vi "ProgrämmschenEinfacherEditor.vi"() -> ()   [LabVIEW 2010]
uses:
  <vilib>/userDefined/High Color/nirio_resource_hc.ctl
  <vilib>/rvi/interface/nirviOpenFPGA/nirviOpenFPGA.xnode
  C:/Users/HAGAR-IV/Desktop/Zeugs/markus/version feb 2012/test/Auslesenkopiekopie2.vi
  <vilib>/rvi/interface/nirviMethod/nirviMethod.xnode
  <vilib>/rvi/interface/nirviReadWriteControl/nirviReadWriteControl.xnode
  <vilib>/rvi/errors/niLvFpgaWhatHappensToTopLevelVI.ctl
  <vilib>/rvi/interface/common/niFpgaNodeNameForErrorReporting.ctl
  <vilib>/rvi/errors/niLvFpgaAdjustHostInterfaceError.vi
  gvbooleschRT.vi
  <vilib>/functionblocks/FB Core/FB Core.xnode
  <vilib>/functionblocks/Counter/Elapsed Timer/Elapsed Timer.vi
  <vilib>/functionblocks/NI_FunctionBlock Libraries.lvlib
  <vilib>/rvi/interface/nirviCloseFPGA/nirviCloseFPGA.xnode
  <vilib>/addons/control/pid/NI_PID_pid.lvlib
  <vilib>/addons/control/pid/pid.llb/PID (DBL).vi
  <vilib>/LabVIEW Targets/FPGA/cRIO/shared/nicrio_ModuleControls/nicrio_cRIO-9871_BaudRateEnum.ctl
  <vilib>/LabVIEW Targets/FPGA/cRIO/shared/nicrio_ModuleControls/nicrio_cRIO-9871_DataBitsEnum.ctl
  <vilib>/LabVIEW Targets/FPGA/cRIO/shared/nicrio_ModuleControls/nicrio_cRIO-9871_ParityEnum.ctl
  <vilib>/LabVIEW Targets/FPGA/cRIO/shared/nicrio_ModuleControls/nicrio_cRIO-9871_StopBitsEnum.ctl
  <vilib>/LabVIEW Targets/FPGA/cRIO/shared/nicrio_ModuleControls/nicrio_cRIO-9871_FlowControlEnum.ctl
  <vilib>/addons/internet/NI_InternetTK_FTP_VIs.lvlib
  <vilib>/RVI Host/nirviSupport.llb/nirviErrorClusterFromErrorCode.vi
  <vilib>/FPGAPlugInAG/cRIO-9114/niLvFpga_Close_cRIO-9114.vi
panel:
  in  "dargestellte Größe 2":i32(ring)=1 items=["T-MainCol3", "T-Trap1", "T-Trap2", "T-Stirling", "T-PreCol1", "T-PreCol2", "T-MainCol1", "T-MainCol2", "T-T-Line2", "T-MI1", "T-MI2", "T-MI3", "T-MI4", "T-MI5", "T-MI6", "F-MFM1", "T-MainCol4", "T-BHorst1", "T-BHorst2", "T-BHorst3", "T-BHorst4", "T-Oven1", "T-Oven2", "T-T-Line1", "F-MFM2", "P-Me-HP", "P-Me-LP", "P-Vac", "Ref-Turbo", "I-MS-AC", "I-Trap1", "I-Trap2", "Mod2/AI0", "Mod2/AI1", "Mod2/AI2", "Mod2/AI3", "Mod2/AI4", "Mod2/AI5", "Mod2/AI6", "Mod2/AI7", "Mod2/AI8", "Mod2/AI9", "Mod2/AI10", "Mod2/AI11", "Mod2/AI12", "Mod2/AI13", "Mod2/AI14", "Mod2/AI15", "Mod2/AI16", "Mod2/AI17", "Mod2/AI18", "Mod2/AI19", "Mod2/AI20", "Mod2/AI21", "Mod2/AI22", "Mod2/AI23", "Mod2/AI24", "Mod2/AI25", "Mod2/AI26", "Mod2/AI27", "Mod2/AI28", "Mod2/AI29", "Mod2/AI30", "Mod2/AI31", "Mod3/AI0", "Mod3/AI1", "Mod3/AI2", "Mod3/AI3", "Mod3/AI4", "Mod3/AI5", "Mod3/AI6", "Mod3/AI7", "Mod3/AI8", "Mod3/AI9", "Mod3/AI10", "Mod3/AI11", "Mod3/AI12", "Mod3/AI13", "Mod3/AI14", "Mod3/AI15", "Mod3/AI16", "Mod3/AI17", "Mod3/AI18", "Mod3/AI19", "Mod3/AI20", "Mod3/AI21", "Mod3/AI22", "Mod3/AI23", "Mod3/AI24", "Mod3/AI25", "Mod3/AI26", "Mod3/AI27", "Mod3/AI28", "Mod3/AI29", "Mod3/AI30", "Mod3/AI31", "U_Widr.Trap1 [V]", "Temp.Trap1 [°C]", "U_Widr.Trap2 [V]", "Temp.Trap2 [°C]", "Temp.Mach1 [°C]", "Temp.Mach2 [°C]", "MFC1B", "PressContr1A", "PressContr1B", "PressContr1C", "MFC1A", "PressContr1D"]
  in  "Zeitachse2":i32(ring)=1 items=["Zykluszeit [s] Mod0", "Zykluszeit [s] Mod1", "Zykluszeit [s] Mod2A", "Zykluszeit [s] Mod2B"]
  out "Anzeige2":cluster{dbl[], dbl[]}(graph)
  out "Datum/Zeit":string
  in  "wie wird gespeichert?":u16(ring) items=["Time", "Cycle", "All"]
  out "Text 6":string
  in  "Info":string
  in  "Speicherlänge":string
  in  "Dateien fürs MS schicken?":bool
  in  "Pfad MS-Datei CRIO":path
  in  "Text0 MS-Datei":string
  out "ZwangsHorst!":cluster{dbl[]}[](array[cluster])
  out "ZwangsHorst?":cluster{bool[]}[](array[cluster])
  out "ZwangsDIO!":cluster{bool[]}[](array[cluster])
  out "ZwangsDIO?":cluster{bool[]}[](array[cluster])
  out "PIDs für \"träge\" Heizungen":T1(array[cluster])
  out "ZwangsLangsameH!":bool[](array[boolean])
  in  "Heizen?LH":bool[](array[boolean])
  out "Zwangsbedingungen":dbl[][](array[numeric])
  out "Traps/Machs":dbl[](array[numeric])
  out "ZwangsFPGABoolesch!":bool[](array[boolean])
  out "ZwangsFPGABoolesch?":bool[](array[boolean])
  in  "LangsameHeizungen%":u32[](array[numeric])
  in  "LangsameHeizungenSP":dbl[](array[numeric])
  out "ZwangsLangsameH?":bool[](array[boolean])
  out "Zykluszeiten 0, 1, 2A, 2B":dbl[](array[numeric])
  out "Zyklusnummern 0, 1, 2A, 2B":i32[](array[numeric])
  in  "dargestellte Größe 1":i32(ring)=1 items=["T-MainCol3", "T-Trap1", "T-Trap2", "T-Stirling", "T-PreCol1", "T-PreCol2", "T-MainCol1", "T-MainCol2", "T-T-Line2", "T-MI1", "T-MI2", "T-MI3", "T-MI4", "T-MI5", "T-MI6", "F-MFM1", "T-MainCol4", "T-BHorst1", "T-BHorst2", "T-BHorst3", "T-BHorst4", "T-Oven1", "T-Oven2", "T-T-Line1", "F-MFM2", "P-Me-HP", "P-Me-LP", "P-Vac", "Ref-Turbo", "I-MS-AC", "I-Trap1", "I-Trap2", "Mod2/AI0", "Mod2/AI1", "Mod2/AI2", "Mod2/AI3", "Mod2/AI4", "Mod2/AI5", "Mod2/AI6", "Mod2/AI7", "Mod2/AI8", "Mod2/AI9", "Mod2/AI10", "Mod2/AI11", "Mod2/AI12", "Mod2/AI13", "Mod2/AI14", "Mod2/AI15", "Mod2/AI16", "Mod2/AI17", "Mod2/AI18", "Mod2/AI19", "Mod2/AI20", "Mod2/AI21", "Mod2/AI22", "Mod2/AI23", "Mod2/AI24", "Mod2/AI25", "Mod2/AI26", "Mod2/AI27", "Mod2/AI28", "Mod2/AI29", "Mod2/AI30", "Mod2/AI31", "Mod3/AI0", "Mod3/AI1", "Mod3/AI2", "Mod3/AI3", "Mod3/AI4", "Mod3/AI5", "Mod3/AI6", "Mod3/AI7", "Mod3/AI8", "Mod3/AI9", "Mod3/AI10", "Mod3/AI11", "Mod3/AI12", "Mod3/AI13", "Mod3/AI14", "Mod3/AI15", "Mod3/AI16", "Mod3/AI17", "Mod3/AI18", "Mod3/AI19", "Mod3/AI20", "Mod3/AI21", "Mod3/AI22", "Mod3/AI23", "Mod3/AI24", "Mod3/AI25", "Mod3/AI26", "Mod3/AI27", "Mod3/AI28", "Mod3/AI29", "Mod3/AI30", "Mod3/AI31", "U_Widr.Trap1 [V]", "Temp.Trap1 [°C]", "U_Widr.Trap2 [V]", "Temp.Trap2 [°C]", "Temp.Mach1 [°C]", "Temp.Mach2 [°C]", "MFC1B", "PressContr1A", "PressContr1B", "PressContr1C", "MFC1A", "PressContr1D"]
  in  "Zeitachse1":i32(ring)=1 items=["Zykluszeit [s] Mod0", "Zykluszeit [s] Mod1", "Zykluszeit [s] Mod2A", "Zykluszeit [s] Mod2B"]
  out "Anzeige1":cluster{dbl[], dbl[]}(graph)
  out "Big Ben, Methodenzeit, Zykluszeit0, Zykluszeit1, Zykluszeit2A, Zykluszeit2B":dbl[](array[numeric])
  out "MWHorst":dbl[](array[numeric])
  out "HorstSP":dbl[](array[numeric])
  out "RS-232":string
  out "Port5":string
  out "Zähler serielle Kommunikation":i32
  out "Port6":string
  out "Port7":string
  out "Port8":string
  out "Mod1Mod2Mod3/AITrapsMachs1Hz":dbl[](array[numeric])
  out "Mod3/AI":dbl[](array[numeric])
  out "Mod2/AI":dbl[](array[numeric])
  out "Mod1/AI":dbl[](array[numeric])
  in  "global stop RT":bool
  out "Big Ben":dbl
  out "Methodenzeit":dbl
  out "Zyklnum1ges":i32
  out "aktuelle TDMS-Datei":refnum<k34>
  in  "Methodennummer":i32(ring) items=["0"]
  out "Methodenwechsel?":bool
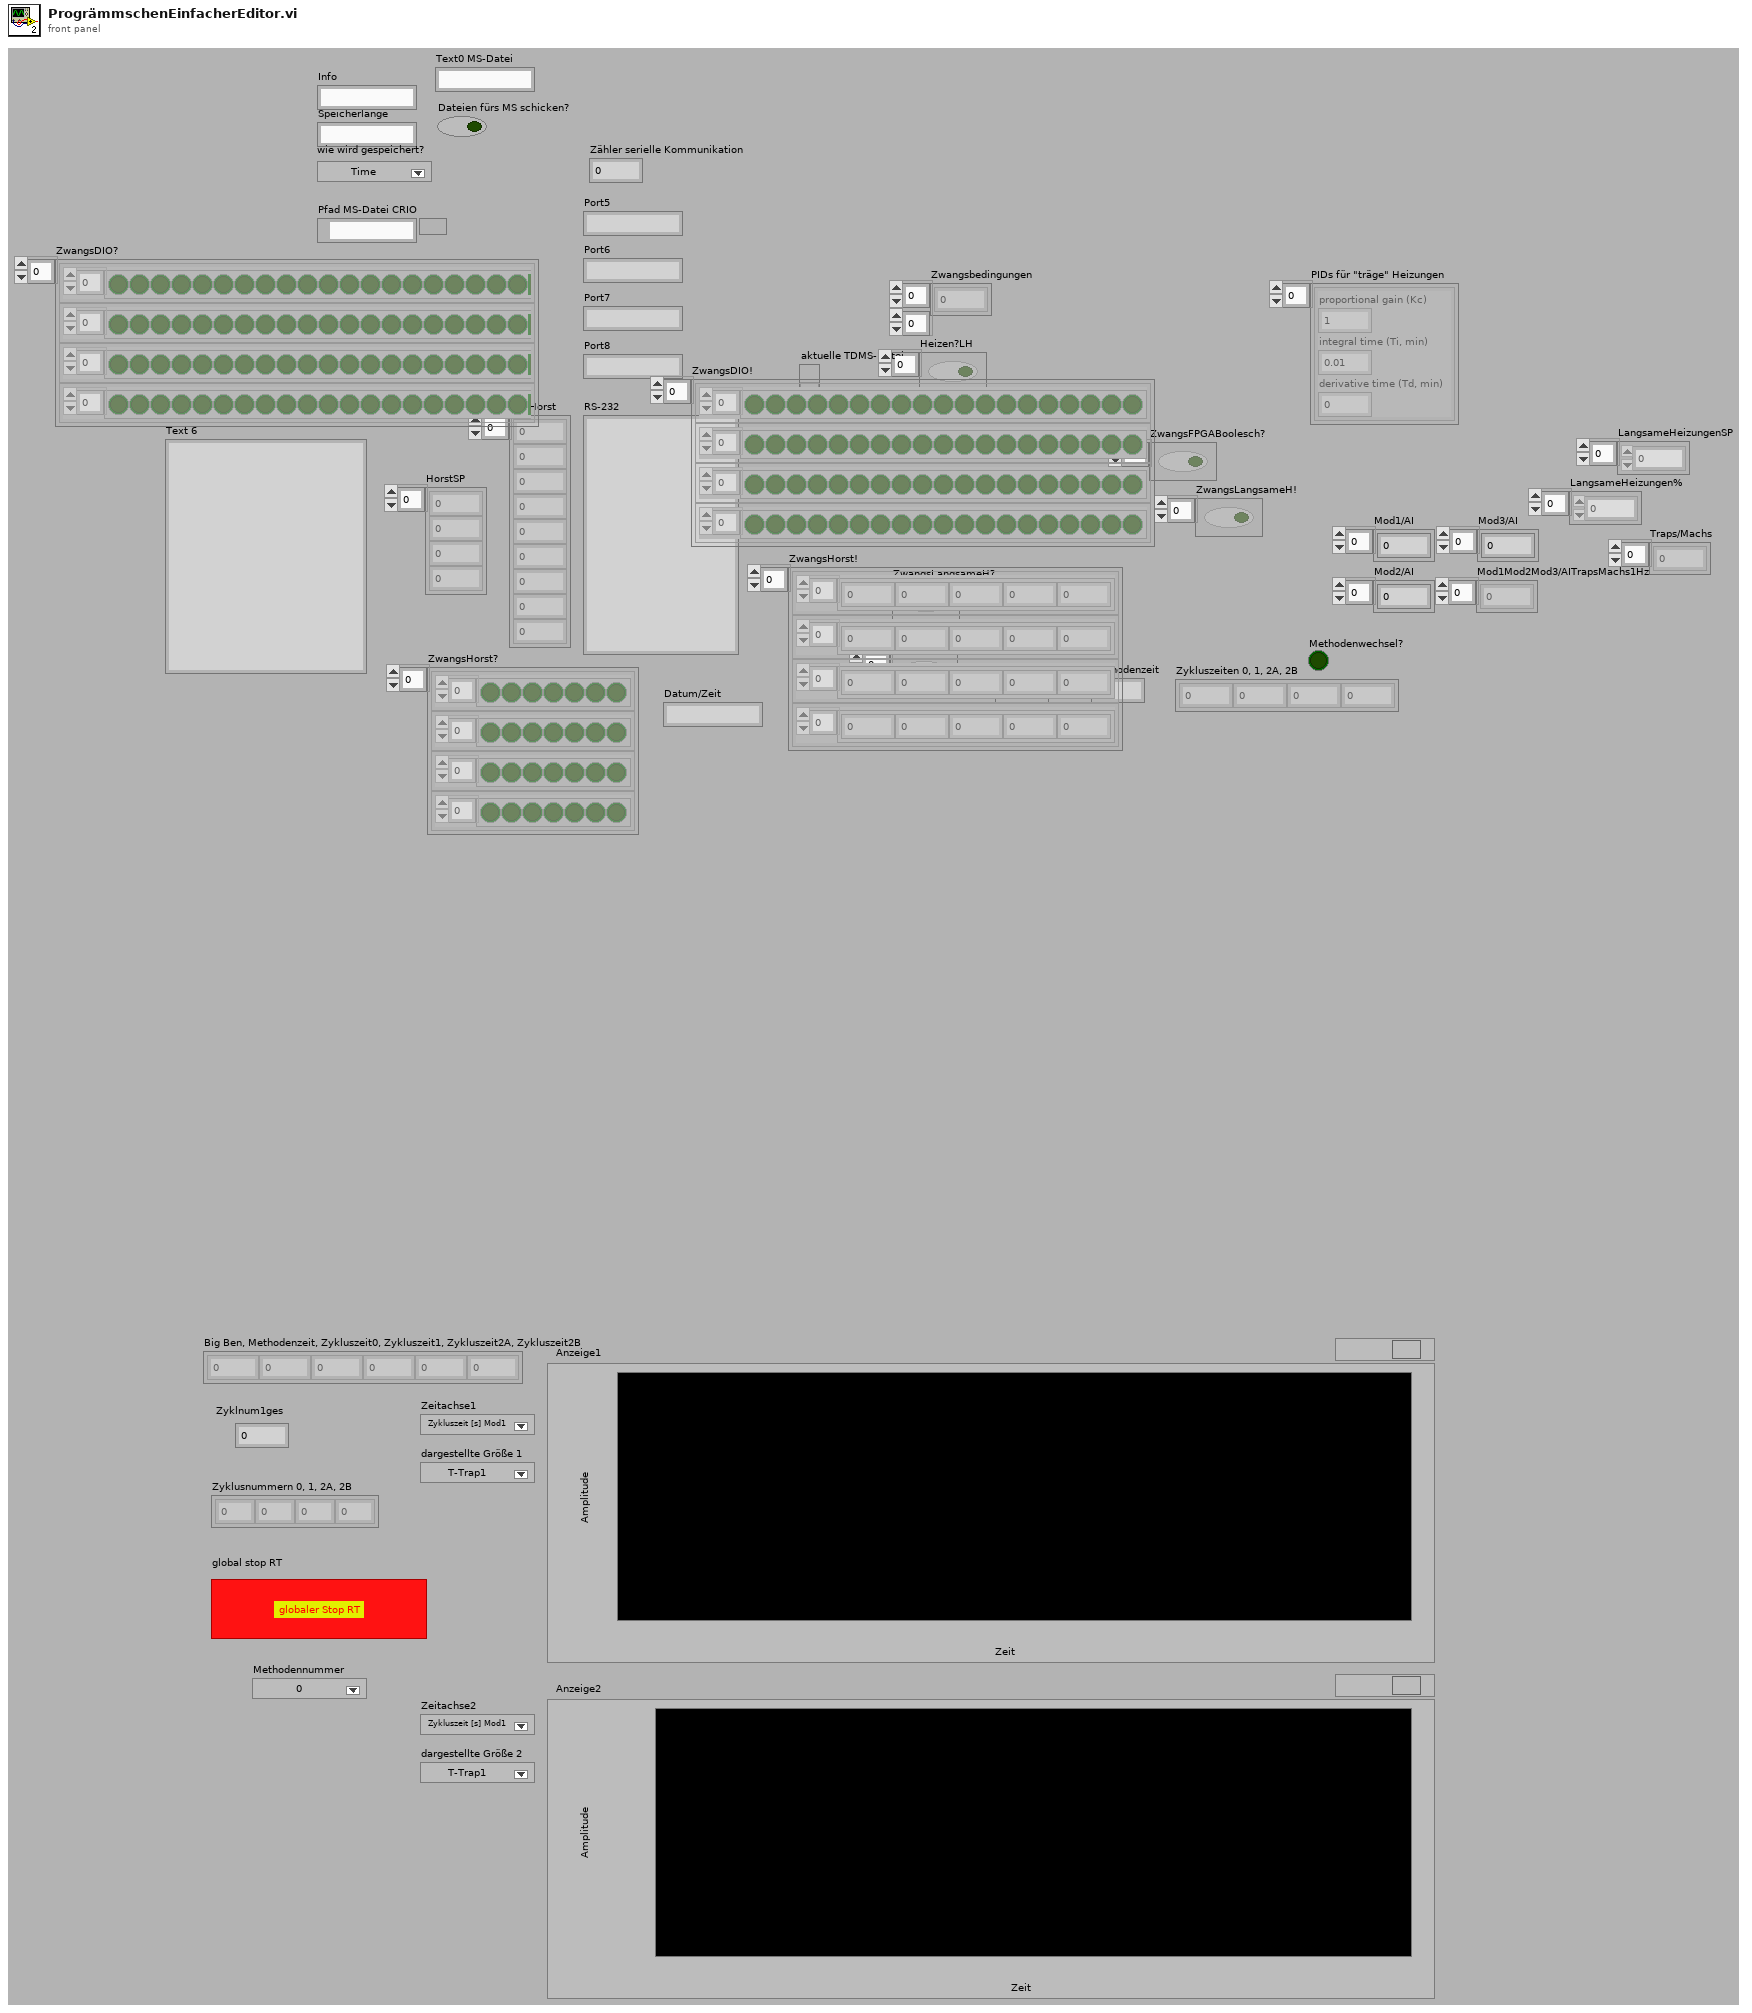
[diagram p1: front panel]
types:
  T1 = cluster{"proportional gain (Kc)":dbl, "integral time (Ti, min)":dbl, "derivative time (Td, min)":dbl}[]
  T2 = cluster{"Zykluslängen [s]":dbl[], "ZeitpktDIOsMod0":dbl[], "ZeitpktDIOsMod1":dbl[], "ZeitpktDIOsMod2A":dbl[], "ZeitpktDIOsMod2B":dbl[], "DIOsSPMod0":bool[][], "DIOsSPMod1":bool[][], "DIOsSPMod2A":bool[][], "DIOsSPMod2B":bool[][], "Mod0HorstZeitpkt":dbl[], "Mod1HorstZeitpkt":dbl[], "Mod2AHorstZeitpkt":dbl[], "Mod2BHorstZeitpkt":dbl[], "HorstSPMod0":dbl[][], "HorstSPMod1":dbl[][], "HorstSPMod2A":dbl[][], "HorstSPMod2B":dbl[][], "LangsameHeizungenSP":dbl[], "LHHeizen?":bool[], "ZPktFPGABoolesch":dbl[], "FPGABoolesch":bool[][], "ZeitpktFPGAPID":dbl[], "FPGAPID":cluster{"proportional gain (Kc)":fxp<+/-,16,8>, "integral gain (Kc*Ts/Ti)":fxp<+/-,16,8>, "derivative gain (Kc*Td/Ts)":fxp<+/-,16,8>}[][], "ZeitpktFPGAFixp":dbl[], "FPGAFixp":fxp<+/-,16,4>[][], "ZeitpktMach1":dbl[], "TempMach1":dbl[], "ZeitpktMach2":dbl[], "TempMach2":dbl[], "PIDs für \"träge\" Heizungen":cluster{"proportional gain (Kc)":dbl, "integral time (Ti, min)":dbl, "derivative time (Td, min)":dbl}[], "Zwangsbedingungen":dbl[][], "Text0 MS-Datei":string, "Info":string, "wie wird gespeichert?":u16, "Speicherlänge":string, "Dateien fürs MS schicken?":bool, "Pfad MS-Datei CRIO":path}[]
  T3 = cluster{"DIOsMod0Nr":i32[], "DIOsMod1Nr":i32[], "DIOsMod2ANr":i32[], "DIOsMod2BNr":i32[], "AIs für \"träge\" Heizungen":i32[], i32[], "AnschlüsseHorstMod0":enum8{"0", "1", "2", "3", "4", "5", "6", "7", "8"}[], "AnschlüsseHorstMod1":enum8{"0", "1", "2", "3", "4", "5", "6", "7", "8"}[], "AnschlüsseHorstMod2A":enum8{"0", "1", "2", "3", "4", "5", "6", "7", "8"}[], "AnschlüsseHorstMod2B":enum8{"0", "1", "2", "3", "4", "5", "6", "7", "8"}[], "StringSPvorgebenMod0":string[], "StringSPvorgebenMod1":string[], "StringSPvorgebenMod2A":string[], "StringSPvorgebenMod2B":string[], "StringMWAntwort0":string[], "StringMWAntwort1":string[], "StringMWAntwort2A":string[], "StringMWAntwort2B":string[], "UmrechnungHorst0":dbl[], "UmrechnungHorst1":dbl[], "UmrechnungHorst2A":dbl[], "UmrechnungHorst2B":dbl[], "StringMWabfragenMod0":string[], "StringMWabfragenMod1":string[], "StringMWabfragenMod2A":string[], "StringMWabfragenMod2B":string[], "Modul1/AI koeff":dbl[][], "Modul2/AI koeff":dbl[][], "Modul3/AI koeff":dbl[][], "Traps/MachKoeff":dbl[][], "AIsNamen":string[], "DIOsMod0Name":string[], "DIOsMod1Name":string[], "DIOsMod2AName":string[], "DIOsMod2BName":string[], "HorstMod0Name":string[], "HorstMod1Name":string[], "HorstMod2AName":string[], "HorstMod2BName":string[], "Startmethode":i32, "Dateiordner Housekeeping":path, "Dateiname Housekeeping":string}
  T4 = enum16{"open", "open or create", "create or replace", "create", "open (read-only)"}
  T5 = enum16{"open", "replace", "create", "open or create", "replace or create", "replace or create with confirmation"}
  T6 = typedef "niFpgaNodeNameForErrorReporting.ctl" = enum16{"Open FPGA VI Reference", "Read/Write Control", "Invoke Method: Abort", "Invoke Method: Acknowledge IRQ", "Invoke Method: Download", "Invoke Method: FIFO.Configure", "Invoke Method: FIFO.Read", "Invoke Method: FIFO.Start", "Invoke Method: FIFO.Stop", "Invoke Method: FIFO.Write", "Invoke Method: Reset", "Invoke Method: Run", "Invoke Method: Wait on IRQ", "Close FPGA VI Reference"}
  T7 = typedef "niLvFpgaWhatHappensToTopLevelVI.ctl" = enum16{"top level VI scripted behind XNode", "top level VI inlined behind XNode"}
  T8 = typedef "nicrio_cRIO-9871_BaudRateEnum.ctl" = enum16{"75 bps", "110 bps", "134 bps", "150 bps", "300 bps", "600 bps", "1200 bps", "1800 bps", "2400 bps", "4800 bps", "7200 bps", "9600 bps", "14.4 kbps", "19.2 kbps", "28.8 kbps", "38.4 kbps", "57.6 kbps", "115.2 kbps", "230.4 kbps", "460.8 kbps", "921.6 kbps"}
  T9 = typedef "nicrio_cRIO-9871_DataBitsEnum.ctl" = enum8{"5", "6", "7", "8"}
  T10 = typedef "nicrio_cRIO-9871_ParityEnum.ctl" = enum8{"None", "Odd", "Even", "Mark", "Space"}
  T11 = typedef "nicrio_cRIO-9871_StopBitsEnum.ctl" = enum8{"1", "1.5", "2"}
  T12 = typedef "nicrio_cRIO-9871_FlowControlEnum.ctl" = enum8{"None", "Software (XON / XOFF)", "Hardware (RTS / CTS)"}
  T13 = cluster{"Baud Rate":T8, "Data Bits":T9, "Parity":T10, "Stop Bits":T11, "Flow Control":T12}
  T14 = enum8{"0", "1", "2", "3", "4", "5", "6", "7", "8"}[]
  T15 = cluster{"Heizen?LH[0]":bool, "Heizen?LH[1]":bool, "Heizen?LH[2]":bool, "Heizen?LH[3]":bool, "Heizen?LH[4]":bool, "Heizen?LH[5]":bool}
  T16 = cluster{"LangsameHeizungen%[0]":u32, "LangsameHeizungen%[1]":u32, "LangsameHeizungen%[2]":u32, "LangsameHeizungen%[3]":u32, "LangsameHeizungen%[4]":u32, "LangsameHeizungen%[5]":u32}
  T17 = cluster{"PIDs für \"träge\" Heizungen[0]":cluster{"proportional gain (Kc)":dbl, "integral time (Ti, min)":dbl, "derivative time (Td, min)":dbl}, "PIDs für \"träge\" Heizungen[1]":cluster{"proportional gain (Kc)":dbl, "integral time (Ti, min)":dbl, "derivative time (Td, min)":dbl}, "PIDs für \"träge\" Heizungen[2]":cluster{"proportional gain (Kc)":dbl, "integral time (Ti, min)":dbl, "derivative time (Td, min)":dbl}, "PIDs für \"träge\" Heizungen[3]":cluster{"proportional gain (Kc)":dbl, "integral time (Ti, min)":dbl, "derivative time (Td, min)":dbl}, "PIDs für \"träge\" Heizungen[4]":cluster{"proportional gain (Kc)":dbl, "integral time (Ti, min)":dbl, "derivative time (Td, min)":dbl}, "PIDs für \"träge\" Heizungen[5]":cluster{"proportional gain (Kc)":dbl, "integral time (Ti, min)":dbl, "derivative time (Td, min)":dbl}}
  T18 = cluster{"LangsameHeizungenSP[0]":dbl, "LangsameHeizungenSP[1]":dbl, "LangsameHeizungenSP[2]":dbl, "LangsameHeizungenSP[3]":dbl, "LangsameHeizungenSP[4]":dbl, "LangsameHeizungenSP[5]":dbl}
  T19 = cluster{"[0]":dbl, "[1]":dbl, "[2]":dbl, "[3]":dbl, "[4]":dbl, "[5]":dbl}
  T20 = cluster{"proportional gain (Kc)":dbl, "integral time (Ti, min)":dbl, "derivative time (Td, min)":dbl}
  T21 = cluster{"Zykluslängen [s]":dbl[], "ZeitpktDIOsMod0":dbl[], "ZeitpktDIOsMod1":dbl[], "ZeitpktDIOsMod2A":dbl[], "ZeitpktDIOsMod2B":dbl[], "DIOsSPMod0":bool[][], "DIOsSPMod1":bool[][], "DIOsSPMod2A":bool[][], "DIOsSPMod2B":bool[][], "Mod0HorstZeitpkt":dbl[], "Mod1HorstZeitpkt":dbl[], "Mod2AHorstZeitpkt":dbl[], "Mod2BHorstZeitpkt":dbl[], "HorstSPMod0":dbl[][], "HorstSPMod1":dbl[][], "HorstSPMod2A":dbl[][], "HorstSPMod2B":dbl[][], "LangsameHeizungenSP":dbl[], "LHHeizen?":bool[], "ZPktFPGABoolesch":dbl[], "FPGABoolesch":bool[][], "ZeitpktFPGAPID":dbl[], "FPGAPID":cluster{"proportional gain (Kc)":fxp<+/-,16,8>, "integral gain (Kc*Ts/Ti)":fxp<+/-,16,8>, "derivative gain (Kc*Td/Ts)":fxp<+/-,16,8>}[][], "ZeitpktFPGAFixp":dbl[], "FPGAFixp":fxp<+/-,16,4>[][], "ZeitpktMach1":dbl[], "TempMach1":dbl[], "ZeitpktMach2":dbl[], "TempMach2":dbl[], "PIDs für \"träge\" Heizungen":cluster{"proportional gain (Kc)":dbl, "integral time (Ti, min)":dbl, "derivative time (Td, min)":dbl}[], "Zwangsbedingungen":dbl[][], "Text0 MS-Datei":string, "Info":string, "wie wird gespeichert?":u16, "Speicherlänge":string, "Dateien fürs MS schicken?":bool, "Pfad MS-Datei CRIO":path}
  T22 = cluster{"proportional gain (Kc)":fxp<+/-,16,8>, "integral gain (Kc*Ts/Ti)":fxp<+/-,16,8>, "derivative gain (Kc*Td/Ts)":fxp<+/-,16,8>}[][]
  T23 = cluster{"FPGAFixp[0]":fxp<+/-,16,4>, "FPGAFixp[1]":fxp<+/-,16,4>, "FPGAFixp[2]":fxp<+/-,16,4>, "FPGAFixp[3]":fxp<+/-,16,4>, "FPGAFixp[4]":fxp<+/-,16,4>, "FPGAFixp[5]":fxp<+/-,16,4>, "FPGAFixp[6]":fxp<+/-,16,4>, "FPGAFixp[7]":fxp<+/-,16,4>}
  T24 = cluster{"proportional gain (Kc)":fxp<+/-,16,8>, "integral gain (Kc*Ts/Ti)":fxp<+/-,16,8>, "derivative gain (Kc*Td/Ts)":fxp<+/-,16,8>}[]
  T25 = cluster{"FPGAPID[0]":cluster{"proportional gain (Kc)":fxp<+/-,16,8>, "integral gain (Kc*Ts/Ti)":fxp<+/-,16,8>, "derivative gain (Kc*Td/Ts)":fxp<+/-,16,8>}, "FPGAPID[1]":cluster{"proportional gain (Kc)":fxp<+/-,16,8>, "integral gain (Kc*Ts/Ti)":fxp<+/-,16,8>, "derivative gain (Kc*Td/Ts)":fxp<+/-,16,8>}, "FPGAPID[2]":cluster{"proportional gain (Kc)":fxp<+/-,16,8>, "integral gain (Kc*Ts/Ti)":fxp<+/-,16,8>, "derivative gain (Kc*Td/Ts)":fxp<+/-,16,8>}, "FPGAPID[3]":cluster{"proportional gain (Kc)":fxp<+/-,16,8>, "integral gain (Kc*Ts/Ti)":fxp<+/-,16,8>, "derivative gain (Kc*Td/Ts)":fxp<+/-,16,8>}}
  T26 = cluster{"proportional gain (Kc)":fxp<+/-,16,8>, "integral gain (Kc*Ts/Ti)":fxp<+/-,16,8>, "derivative gain (Kc*Td/Ts)":fxp<+/-,16,8>}
  T27 = cluster{"[0]":bool, "[1]":bool, "[2]":bool, "[3]":bool, "[4]":bool, "[5]":bool}
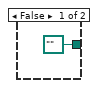
[diagram p2: hidden frame]
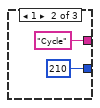
[diagram p4: hidden frame]
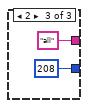
[diagram p5: hidden frame]
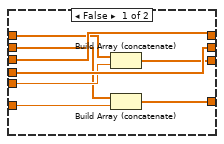
[diagram p9: hidden frame]
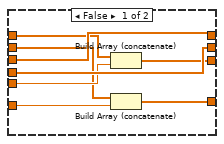
[diagram p10: hidden frame]
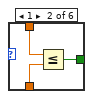
[diagram p14: hidden frame]
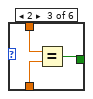
[diagram p15: hidden frame]
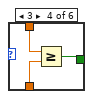
[diagram p16: hidden frame]
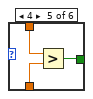
[diagram p17: hidden frame]
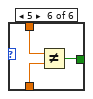
[diagram p18: hidden frame]
diagram:
  w1 = T2 [{"Zykluslängen [s]"=[10.0, 60.0, 10.0, 10.0], "ZeitpktDIOsMod0"=[0.0, 10.0], "ZeitpktDIOsMod1"=[0.0, 60.0], "ZeitpktDIOsMod2A"=[0.0, 10.0], "ZeitpktDIOsMod2B"=[0.0, 10.0], "DIOsSPMod0"=[[FALSE], [FALSE]], "DIOsSPMod1"=[[FALSE, FALSE, FALSE, FALSE, FALSE, FALSE, FALSE, FALSE, FALSE, FALSE, FALSE, FALSE, FALSE, FALSE, FALSE, FALSE, FALSE, FALSE], [FALSE, FALSE, FALSE, FALSE, FALSE, FALSE, FALSE, FALSE, FALSE, FALSE, FALSE, FALSE, FALSE, FALSE, FALSE, FALSE, FALSE, FALSE]], "DIOsSPMod2A"=[[FALSE], [FALSE]], "DIOsSPMod2B"=[[FALSE], [FALSE]], "Mod0HorstZeitpkt"=[0.0, 10.0], "Mod1HorstZeitpkt"=[0.0, 60.0], "Mod2AHorstZeitpkt"=[0.0, 10.0], "Mod2BHorstZeitpkt"=[0.0, 10.0], "HorstSPMod0"=[[0.0], [0.0]], "HorstSPMod1"=[[0.0, 0.0, 0.0], [0.0, 0.0, 0.0]], "HorstSPMod2A"=[[0.0], [0.0]], "HorstSPMod2B"=[[0.0], [0.0]], "LangsameHeizungenSP"=[0.0, 0.0, 0.0, 0.0, 0.0, 0.0], "LHHeizen?"=[FALSE, FALSE, FALSE, FALSE, FALSE, FALSE], "ZPktFPGABoolesch"=[0.0, 5.0, 15.0, 17.0, 60.0], "FPGABoolesch"=[[TRUE, FALSE, FALSE, FALSE, FALSE, FALSE], [FALSE, FALSE, TRUE, FALSE, FALSE, FALSE], [FALSE, FALSE, FALSE, FALSE, FALSE, FALSE], [TRUE, FALSE, FALSE, FALSE, FALSE, FALSE], [FALSE, FALSE, FALSE, FALSE, FALSE, FALSE]], "ZeitpktFPGAPID"=[0.0, 60.0], "FPGAPID"=[[{"proportional gain (Kc)"=1.0, "integral gain (Kc*Ts/Ti)"=1.66796875, "derivative gain (Kc*Td/Ts)"=0.0}, {"proportional gain (Kc)"=1.0, "integral gain (Kc*Ts/Ti)"=1.66796875, "derivative gain (Kc*Td/Ts)"=0.0}, {"proportional gain (Kc)"=1.0, "integral gain (Kc*Ts/Ti)"=1.66796875, "derivative gain (Kc*Td/Ts)"=0.0}, {"proportional gain (Kc)"=1.0, "integral gain (Kc*Ts/Ti)"=1.66796875, "derivative gain (Kc*Td/Ts)"=0.0}], [{"proportional gain (Kc)"=1.0, "integral gain (Kc*Ts/Ti)"=1.66796875, "derivative gain (Kc*Td/Ts)"=0.0}, {"proportional gain (Kc)"=1.0, "integral gain (Kc*Ts/Ti)"=1.66796875, "derivative gain (Kc*Td/Ts)"=0.0}, {"proportional gain (Kc)"=1.0, "integral gain (Kc*Ts/Ti)"=1.66796875, "derivative gain (Kc*Td/Ts)"=0.0}, {"proportional gain (Kc)"=1.0, "integral gain (Kc*Ts/Ti)"=1.66796875, "derivative gain (Kc*Td/Ts)"=0.0}]], "ZeitpktFPGAFixp"=[0.0, 60.0], "FPGAFixp"=[[3.5, 3.60009765625, 2.0, 0.0, 0.0, 0.0, 0.0, 0.0], [3.5, 3.60009765625, 2.0, 0.0, 0.0, 0.0, 0.0, 0.0]], "ZeitpktMach1"=[0.0, 60.0], "TempMach1"=[0.0, 0.0], "ZeitpktMach2"=[0.0, 60.0], "TempMach2"=[0.0, 0.0], "PIDs für \"träge\" Heizungen"=[{"proportional gain (Kc)"=1.0, "integral time (Ti, min)"=0.01, "derivative time (Td, min)"=0.0}, {"proportional gain (Kc)"=1.0, "integral time (Ti, min)"=0.01, "derivative time (Td, min)"=0.0}, {"proportional gain (Kc)"=1.0, "integral time (Ti, min)"=0.01, "derivative time (Td, min)"=0.0}, {"proportional gain (Kc)"=1.0, "integral time (Ti, min)"=0.01, "derivative time (Td, min)"=0.0}, {"proportional gain (Kc)"=1.0, "integral time (Ti, min)"=0.01, "derivative time (Td, min)"=0.0}, {"proportional gain (Kc)"=1.0, "integral time (Ti, min)"=0.01, "derivative time (Td, min)"=0.0}], "Zwangsbedingungen"=[[0.0, 0.0, 0.0, 0.0, 0.0]], "Text0 MS-Datei"="text0", "Info"="info", "wie wird gespeichert?"=0, "Speicherlänge"="100", "Dateien fürs MS schicken?"=FALSE, "Pfad MS-Datei CRIO"=path "c:/"}] ("Zykluszeug")
  n1 = flat-sequence {
    tunnel: [w101] -> w31
    tunnel: [w34] -> w30
    tunnel: [w113] -> w29
    tunnel: [w114] -> w28
    tunnel: [w100] -> w24
    tunnel: [w77] -> w23
    tunnel: [w43] -> w22
    tunnel: [w91] -> w21
    tunnel: [w55] -> w20
    tunnel: [w82] -> w19
    tunnel: [w76] -> w18
    tunnel: [w75] -> w17
    tunnel: [w74] -> w16
    tunnel: [w97] -> w15
    tunnel: [w73] -> w14
    tunnel: [w48] -> w13
    tunnel: [w42] -> w12
    tunnel: [w54] -> w11
    tunnel: [w99] -> w10
    tunnel: [w96] -> w9
    tunnel: [w96] -> w8
    tunnel: T3 {"DIOsMod0Nr"=[32], "DIOsMod1Nr"=[5, 6, 7, 10, 11, 14, 15, 16, 17, 18, 20, 23, 25, 26, 27, 28, 29, 30], "DIOsMod2ANr"=[33], "DIOsMod2BNr"=[34], "AIs für \"träge\" Heizungen"=[17, 6, 0, 19, 21, 23], [1, 3, 1, 1], "AnschlüsseHorstMod0"=[enum."1"], "AnschlüsseHorstMod1"=[enum."1", enum."1", enum."1"], "AnschlüsseHorstMod2A"=[enum."1"], "AnschlüsseHorstMod2B"=[enum."1"], "StringSPvorgebenMod0"=[":060A020121"], "StringSPvorgebenMod1"=[":060B020121", ":0618020121", ":060D020121"], "StringSPvorgebenMod2A"=[":0619020121"], "StringSPvorgebenMod2B"=[":060C020121"], "StringMWAntwort0"=[":060A020121"], "StringMWAntwort1"=[":060B020121", ":0618020121", ":060D020121"], "StringMWAntwort2A"=[":0619020121"], "StringMWAntwort2B"=[":060C020121"], "UmrechnungHorst0"=[0.0003125], "UmrechnungHorst1"=[9.375e-05, 9.375e-05, 9.375e-05], "UmrechnungHorst2A"=[0.046875], "UmrechnungHorst2B"=[9.375e-05], "StringMWabfragenMod0"=[":060A0401210120"], "StringMWabfragenMod1"=[":060B0401210120", ":06180401210120", ":060D0401210120"], "StringMWabfragenMod2A"=[":06190401210120"], "StringMWabfragenMod2B"=[":060C0401210120"], "Modul1/AI koeff"=[[-249.333, 111.873, 2.1471], [-249.333, 111.873, 2.1471], [-249.333, 111.873, 2.1471], [-249.333, 111.873, 2.1471], [-237.2852, -153.162, 6.0782], [-237.2852, -153.162, 6.0782], [-249.333, 111.873, 2.1471], [-249.333, 111.873, 2.1471], [-249.333, 111.873, 2.1471], [-249.333, 111.873, 2.1471], [-249.333, 111.873, 2.1471], [-249.333, 111.873, 2.1471], [-249.333, 111.873, 2.1471], [-249.333, 111.873, 2.1471], [-249.333, 111.873, 2.1471], [0.0, 1.0, 0.0], [-249.333, 111.873, 2.1471], [-249.333, 111.873, 2.1471], [-249.333, 111.873, 2.1471], [-249.333, 111.873, 2.1471], [-249.333, 111.873, 2.1471], [-249.333, 111.873, 2.1471], [-249.333, 111.873, 2.1471], [-249.333, 111.873, 2.1471], [0.0, 1.0, 0.0], [0.0, 1.0, 0.0], [0.0, 1.0, 0.0], [0.0, 1.0, 0.0], [0.0, 1.0, 0.0], [0.0, 1.0, 0.0], [0.0, 1.0, 0.0], [0.0, 1.0, 0.0]], "Modul2/AI koeff"=[[0.0, 1.0, 0.0], [0.0, 1.0, 0.0], [0.0, 1.0, 0.0], [0.0, 1.0, 0.0], [0.0, 1.0, 0.0], [0.0, 1.0, 0.0], [0.0, 1.0, 0.0], [0.0, 1.0, 0.0], [0.0, 1.0, 0.0], [0.0, 1.0, 0.0], [0.0, 1.0, 0.0], [0.0, 1.0, 0.0], [0.0, 1.0, 0.0], [0.0, 1.0, 0.0], [0.0, 1.0, 0.0], [0.0, 1.0, 0.0], [0.0, 1.0, 0.0], [0.0, 1.0, 0.0], [0.0, 1.0, 0.0], [0.0, 1.0, 0.0], [0.0, 1.0, 0.0], [0.0, 1.0, 0.0], [0.0, 1.0, 0.0], [0.0, 1.0, 0.0], [0.0, 1.0, 0.0], [0.0, 1.0, 0.0], [0.0, 1.0, 0.0], [0.0, 1.0, 0.0], [0.0, 1.0, 0.0], [0.0, 1.0, 0.0], [0.0, 1.0, 0.0], [0.0, 1.0, 0.0]], "Modul3/AI koeff"=[[0.0, 1.0, 0.0], [0.0, 1.0, 0.0], [0.0, 1.0, 0.0], [0.0, 1.0, 0.0], [0.0, 1.0, 0.0], [0.0, 1.0, 0.0], [0.0, 1.0, 0.0], [0.0, 1.0, 0.0], [0.0, 1.0, 0.0], [0.0, 1.0, 0.0], [0.0, 1.0, 0.0], [0.0, 1.0, 0.0], [0.0, 1.0, 0.0], [0.0, 1.0, 0.0], [0.0, 1.0, 0.0], [0.0, 1.0, 0.0], [0.0, 1.0, 0.0], [0.0, 1.0, 0.0], [0.0, 1.0, 0.0], [0.0, 1.0, 0.0], [0.0, 1.0, 0.0], [0.0, 1.0, 0.0], [0.0, 1.0, 0.0], [0.0, 1.0, 0.0], [0.0, 1.0, 0.0], [0.0, 1.0, 0.0], [0.0, 1.0, 0.0], [0.0, 1.0, 0.0], [0.0, 1.0, 0.0], [0.0, 1.0, 0.0], [0.0, 1.0, 0.0], [0.0, 1.0, 0.0]], "Traps/MachKoeff"=[[0.0, 1.0, 0.0], [-249.333, 111.873, 2.1471], [0.0, 1.0, 0.0], [-249.333, 111.873, 2.1471], [-237.2852, 153.1621, 6.0782], [-237.2852, 153.1621, 6.0782]], "AIsNamen"=["T-MainCol3", "T-Trap1", "T-Trap2", "T-Stirling", "T-PreCol1", "T-PreCol2", "T-MainCol1", "T-MainCol2", "T-T-Line2", "T-MI1", "T-MI2", "T-MI3", "T-MI4", "T-MI5", "T-MI6", "F-MFM1", "T-MainCol4", "T-BHorst1", "T-BHorst2", "T-BHorst3", "T-BHorst4", "T-Oven1", "T-Oven2", "T-T-Line1", "F-MFM2", "P-Me-HP", "P-Me-LP", "P-Vac", "Ref-Turbo", "I-MS-AC", "I-Trap1", "I-Trap2", "Mod2/AI0", "Mod2/AI1", "Mod2/AI2", "Mod2/AI3", "Mod2/AI4", "Mod2/AI5", "Mod2/AI6", "Mod2/AI7", "Mod2/AI8", "Mod2/AI9", "Mod2/AI10", "Mod2/AI11", "Mod2/AI12", "Mod2/AI13", "Mod2/AI14", "Mod2/AI15", "Mod2/AI16", "Mod2/AI17", "Mod2/AI18", "Mod2/AI19", "Mod2/AI20", "Mod2/AI21", "Mod2/AI22", "Mod2/AI23", "Mod2/AI24", "Mod2/AI25", "Mod2/AI26", "Mod2/AI27", "Mod2/AI28", "Mod2/AI29", "Mod2/AI30", "Mod2/AI31", "Mod3/AI0", "Mod3/AI1", "Mod3/AI2", "Mod3/AI3", "Mod3/AI4", "Mod3/AI5", "Mod3/AI6", "Mod3/AI7", "Mod3/AI8", "Mod3/AI9", "Mod3/AI10", "Mod3/AI11", "Mod3/AI12", "Mod3/AI13", "Mod3/AI14", "Mod3/AI15", "Mod3/AI16", "Mod3/AI17", "Mod3/AI18", "Mod3/AI19", "Mod3/AI20", "Mod3/AI21", "Mod3/AI22", "Mod3/AI23", "Mod3/AI24", "Mod3/AI25", "Mod3/AI26", "Mod3/AI27", "Mod3/AI28", "Mod3/AI29", "Mod3/AI30", "Mod3/AI31"], "DIOsMod0Name"=["blindDIO0"], "DIOsMod1Name"=["on/off P-MS", "MS Start", "MS Stop", "FanMach1", "FanReserve", "Valve1A", "on/off PrePump", "S1Reserve", "on/off VacP2", "on/off VacP1", "S1D", "FanMach2", "S1C", "on/off Stirling", "S1B", "S1A", "Valve1B", "on/off Turbo"], "DIOsMod2AName"=["blindDIO2A"], "DIOsMod2BName"=["blindDIO2B"], "HorstMod0Name"=["MFC1B"], "HorstMod1Name"=["PressContr1A", "PressContr1B", "PressContr1C"], "HorstMod2AName"=["MFC1A"], "HorstMod2BName"=["PressContr1D"], "Startmethode"=0, "Dateiordner Housekeeping"=path "C:/", "Dateiname Housekeeping"="test"} ("Einstellungen") -> [w98]
    tunnel: [w68] -> w7
    tunnel: w1 -> [w58]
    tunnel: [w53] -> w6
    tunnel: [w35] -> w5
    tunnel: [w33] -> w3
    tunnel: [w32] -> w2
    tunnel: w31 -> [w367]
    tunnel: w30 -> [w401]
    tunnel: w29 -> [w400]
    tunnel: w28 -> [w399]
    tunnel: [w397] -> w27
    tunnel: [w396] -> w26
    tunnel: [w367] -> w25
    tunnel: w24 -> [_]
    tunnel: w23 -> [w375]
    tunnel: w22 -> [w374]
    tunnel: w21 -> [w373]
    tunnel: w20 -> [w372]
    tunnel: w19 -> [w371]
    tunnel: w18 -> [w370]
    tunnel: w17 -> [w369]
    tunnel: w16 -> [w368]
    tunnel: w15 -> [w364]
    tunnel: w14 -> [w360]
    tunnel: w13 -> [w356]
    tunnel: w12 -> [w344]
    tunnel: w11 -> [w353]
    tunnel: w10 -> [w348]
    tunnel: w9 -> [w351]
    tunnel: w8 -> [w350]
    tunnel: w1 -> [w345]
    tunnel: w7 -> [w342]
    tunnel: w6 -> [w341]
    tunnel: w5 -> [w338]
    tunnel: w3 -> [w337]
    tunnel: w2 -> [w336]
    tunnel: w27 -> [w2031]
    tunnel: w26 -> [w2030]
    tunnel: w25 -> [w2029]
    frame #0 {
      w61 = string[] ["U_Widr.Trap1 [V]", "Temp.Trap1 [°C]", "U_Widr.Trap2 [V]", "Temp.Trap2 [°C]", "Temp.Mach1 [°C]", "Temp.Mach2 [°C]"]
      w65 = string[] ["Big Ben [s]", "Methodenzeit [s]", "Zykluszeit [s] Mod0", "Zykluszeit [s] Mod1", "Zykluszeit [s] Mod2A", "Zykluszeit [s] Mod2B"]
      w99 = 6  # AnzahlLH
      w67 = FALSE ("Undefinierte Werte möglich")
      w111 = T13 {"Baud Rate"=enum."38.4 kbps", "Data Bits"=enum."8", "Parity"=enum."None", "Stop Bits"=enum."1", "Flow Control"=enum."None"} ("Port-Einstellungen 2")
      w117 = "z"
      w119 = "m"
      w120 = ".tdms" ("String")
      n2 = global write "gvbooleschRT.vi" "global stop RT"(FALSE ("global stop RT")) -> ()
      n3 = property on="Zeitachse1" class="Ring (strict)"("AllowUndefVals"=w67) -> ()  [unwired: 2 in, 2 out]
      n4 = property on="dargestellte Größe 1" class="Ring (strict)"("AllowUndefVals"=w67) -> ()  [unwired: 2 in, 2 out]
      n5 = property on="Methodennummer" class="Ring (strict)"("AllowUndefVals"=w67) -> ()  [unwired: 2 in, 2 out]
      n6 = Array Size(array=w58) -> (size(s)=w57:i32)
      n7 = for {
        N: w57 -> [_]
        tunnel: [w162] -> w56 mode=indexing
        i -> [w163]
        n8 = Number To Decimal String(number=w163) -> (decimal integer string=w162:string)  [unwired: 1 in]
      }
      n9 = case shown="True" "Dateien fürs MS schicken?" {
        tunnel: [path "" ("path") w149] -> w35
        frame False {
        }
        frame True {
          n10 = Open/Create/Replace File(file path (use dialog)="Pfad MS-Datei CRIO", operation (0:open)=T5."replace or create" ("Operation (0:Öffnen)")) -> (refnum out=w158:refnum<file>, error out=w157:errorcluster)  [unwired: 4 in, 1 out]
          n11 = Open/Create/Replace File(file path (use dialog)=path "c:/fromcriordy.txt" ("Dateipfad (Dialog verwenden)"), operation (0:open)=T5."replace or create" ("Operation (0:Öffnen)")) -> (refnum out=w152:refnum<file>, error out=w153:errorcluster)  [unwired: 4 in, 1 out]
          n12 = Write to Text File(file (use dialog)=w158, text="Text0 MS-Datei", error in=w157) -> (refnum out=w155:refnum<file>, error out=w154:errorcluster)  [unwired: 1 in, 1 out]
          n13 = Close File(refnum=w152, error in=w153) -> (path=w149:path)  [unwired: 1 out]
          n14 = Close File(refnum=w155, error in=w154) -> ()  [unwired: 2 out]
        }
      }
      n15 = xnode "Open FPGA VI Reference"() -> ("FPGA VI Reference Out"=w146:refnum<k20>, "error out"=w147:errorcluster)  [unwired: 2 in]
      n16 = xnode "Invoke Method"("FPGA VI Reference In"=w146, "error in"=w147) -> ("FPGA VI Reference Out"=w145:refnum<k20>, "error out"=w144:errorcluster)
      n17 = property on="Methodennummer" class="Ring (strict)"("Strings []"=w56) -> ()  [unwired: 2 in, 2 out]
      n18 = Number To Decimal String(number=0 ("Wert")) -> (decimal integer string=w121:string)  [unwired: 1 in]
      n19 = Number To Decimal String(number=1 ("Wert")) -> (decimal integer string=w116:string)  [unwired: 1 in]
      n20 = xnode "Read/Write Control"("FPGA VI Reference In"=w145, "error in"=w144, "vor der Messung [us]Mach"=u16 600 ("vor der Messung [us]Mach1"), "wie viele Messwerte?Mach"=u16 14 ("wie viele Messwerte?Mach1"), "Abstand zwischen Messungen [us]Mach"=u16 150 ("Abstand zwischen Messungen [us]Mach1"), "Heizen?Trap1"=FALSE, "Heizen?Trap2"=FALSE, "warten[us]Trap1"=u32 2000, "warten[us]Trap2"=u32 2000, "Per[us]Trap1"=u32 10000, "Per[us]Trap2"=u32 10000, "global stop"=FALSE, "Per[us]Mach"=u16 20000 ("Per[us]Mach1"), "Heizen?Mach1"=FALSE, "Heizen?Mach2"=FALSE, "Port 1"=w111, "Port 2"=w111, "Port 3"=w111, "Port 4"=w111, "Port 5"=w111, "Port 6"=w111, "Port 7"=w111, "Port 8"=w111, "ServosPeriode(us)"=u32 20000, "Servo1WarmHigh(us)"=u32 1430, "Servo1KaltHigh(us)"=u32 1630, "Servo2WarmHigh(us)"=u32 1320, "Servo2KaltHigh(us)"=u32 1520) -> ("FPGA VI Reference Out"=w143:refnum<k20>, "error out"=w142:errorcluster)
      n21 = xnode "Invoke Method"("FPGA VI Reference In"=w143, "error in"=w142) -> ("FPGA VI Reference Out"=w110:refnum<k20>, "error out"=w103:errorcluster)  [unwired: 1 in]
      n22 = Unbundle(w98) -> ("DIOsMod0Nr"=w52:i32[], "DIOsMod1Nr"=w51:i32[], "DIOsMod2ANr"=w50:i32[], "DIOsMod2BNr"=w49:i32[], "AIs für \"träge\" Heizungen"=w97:i32[], w96:i32[], "AnschlüsseHorstMod0"=w47:T14, "AnschlüsseHorstMod1"=w46:T14, "AnschlüsseHorstMod2A"=w45:T14, "AnschlüsseHorstMod2B"=w44:T14, "StringSPvorgebenMod0"=w95:string[], "StringSPvorgebenMod1"=w94:string[], "StringSPvorgebenMod2A"=w93:string[], "StringSPvorgebenMod2B"=w92:string[], "StringMWAntwort0"=w90:string[], "StringMWAntwort1"=w89:string[], "StringMWAntwort2A"=w88:string[], "StringMWAntwort2B"=w87:string[], "UmrechnungHorst0"=w86:dbl[], "UmrechnungHorst1"=w85:dbl[], "UmrechnungHorst2A"=w84:dbl[], "UmrechnungHorst2B"=w83:dbl[], "StringMWabfragenMod0"=w81:string[], "StringMWabfragenMod1"=w80:string[], "StringMWabfragenMod2A"=w79:string[], "StringMWabfragenMod2B"=w78:string[], "Modul1/AI koeff"=w76:dbl[][], "Modul2/AI koeff"=w75:dbl[][], "Modul3/AI koeff"=w74:dbl[][], "Traps/MachKoeff"=w73:dbl[][], "AIsNamen"=w62:string[], "HorstMod0Name"=w72:string[], "HorstMod1Name"=w71:string[], "HorstMod2AName"=w70:string[], "HorstMod2BName"=w69:string[], "Startmethode"=w34:i32, "Dateiordner Housekeeping"=w32:path, "Dateiname Housekeeping"=w33:string)  [unwired: 4 out]
      n23 = property on="Methodennummer" class="Ring (strict)"("Value"=w34) -> ()  [unwired: 2 in, 2 out]
      n24 = Number To Decimal String(number=w34) -> (decimal integer string=w118:string)  [unwired: 1 in]
      n25 = Concatenate Strings(w33, w119, w118, w117, w121, w120) -> (w125:string)
      n26 = Concatenate Strings(w33, w119, w118, w117, w116, w120) -> (w124:string)
      n27 = Build Path(base path=w32, name or relative path=w125) -> (appended path=w126:path)
      n28 = Build Path(base path=w32, name or relative path=w124) -> (appended path=w115:path)
      n29 = Build Array (concatenate)(w47, w46, w45, w44) -> (w43:T14)
      n30 = Build Array (concatenate)(w72, w71, w70, w69) -> (w60:string[])
      n31 = Build Array (concatenate)(w95, w94, w93, w92) -> (w91:string[])
      n32 = TDMS Open(10:T4."create" ("Operation (0:Öffnen)"), 11:w126) -> (3:w113:refnum<k34>)  [unwired: 4 in, 1 out]
      n33 = xnode "Read/Write Control"("FPGA VI Reference In"=w110, "error in"=w103, "Update Config"=TRUE) -> ("FPGA VI Reference Out"=w105:refnum<k20>, "error out"=w102:errorcluster)
      n34 = Build Array (concatenate)(w81, w80, w79, w78) -> (w77:string[])
      n35 = Build Array (concatenate)(w90, w89, w88, w87) -> (w82:string[])
      n36 = local write "aktuelle TDMS-Datei"(w113) -> ()
      n37 = Add Array Elements(numeric array=w96) -> (sum=w54:i32)
      n38 = Build Array (concatenate)(w86, w85, w84, w83) -> (w55:dbl[])
      n39 = xnode "Invoke Method"("FPGA VI Reference In"=w105, "error in"=w102, "Number of Elements"=u32 0) -> ("FPGA VI Reference Out"=w104:refnum<k20>, "error out"=w108:errorcluster, "Elements Remaining"=w106:u32)  [unwired: 1 in, 1 out]
      n40 = Split 1D Array(array=w65, index=2 ("Index")) -> (second subarray=w63:string[])  [unwired: 1 out]
      n41 = property on="Zeitachse1" class="Ring (strict)"("Strings []"=w63) -> ()  [unwired: 2 in, 2 out]
      n42 = Build Array (concatenate)(w62, w61, w60) -> (w59:string[])
      n43 = Build Cluster Array(w52, w51, w50, w49) -> (w48:cluster{"DIOsMod2BNr":i32[]}[])
      n44 = for {
        tunnel: w48 -> [w165] mode=indexing
        tunnel: [w166] -> w42 mode=indexing
        n45 = Unbundle(w165) -> ("DIOsMod2BNr"=w164:i32[])
        n46 = Array Size(array=w164) -> (size(s)=w166:i32)
      }
      n47 = property on="dargestellte Größe 1" class="Ring (strict)"("Strings []"=w59) -> ()  [unwired: 2 in, 2 out]
      n48 = xnode "Invoke Method"("FPGA VI Reference In"=w104, "error in"=w108, "Number of Elements"=w106) -> ("FPGA VI Reference Out"=w101:refnum<k20>, "error out"=w100:errorcluster)  [unwired: 1 in, 2 out]
      n49 = Build Array (concatenate)(string[] ["Datei Nr.", "Zyklusnr. Mod0", "Zyklusnr. Mod1", "Zyklusnr. Mod2A", "Zyklusnr. Mod2B"], w65, w62, w61, w60) -> (w68:string[])
      n50 = TDMS Open(10:T4."create" ("Operation (0:Öffnen)"), 11:w115) -> (3:w114:refnum<k34>)  [unwired: 4 in, 1 out]
      n51 = for {
        N: w54 -> [_]
        tunnel: [0.0] -> w53 mode=indexing
      }
    }
    frame #1 {
      w335 = dbl[] []
      n52 = while {
        shift-right: ["Methodennummer"] -> _
        shift-left: w401 -> [w2024]
        stop <- w2026 stop-if-true
        n53 = call "Warten"("Count(mSec)"=u32 1000) -> ()  [unwired: 1 out]
        n54 = Not Equal?(x=w2024, y="Methodennummer") -> (x != y?=→"Methodenwechsel?":bool)
        n55 = global read "gvbooleschRT.vi" "global stop RT"() -> (w2026:bool)
      }
      n56 = while "\"langsame\" Pulse" {
        tunnel: w367 -> [w691]
        stop <- w692 stop-if-true
        n57 = Array To Cluster(array="Heizen?LH") -> (cluster=w662:T15)
        n58 = Unbundle(w662) -> ("Heizen?LH[0]"=w661:bool, "Heizen?LH[1]"=w660:bool, "Heizen?LH[2]"=w659:bool, "Heizen?LH[3]"=w658:bool, "Heizen?LH[4]"=w657:bool, "Heizen?LH[5]"=w656:bool)
        n59 = xnode "Read/Write Control"("FPGA VI Reference In"=w691, "on/off Bronkhorst I Heater"=w661, "on/off Main-Col I Heater"=w660, "on/off Main-Col II Heater"=w659, "on/off Bronkhorst II Heater"=w658, "on/off Oven Heater"=w657, "on/off T-Line Heater"=w656) -> ("FPGA VI Reference Out"=w672:refnum<k20>)  [unwired: 1 in, 1 out]
        n60 = Array To Cluster(array="LangsameHeizungen%") -> (cluster=w670:T16)
        n61 = Unbundle "Horst1\nMainCol1\nMainCol2\nHorst2\nOven\nT-Line"(w670) -> ("LangsameHeizungen%[0]"=w669:u32, "LangsameHeizungen%[1]"=w668:u32, "LangsameHeizungen%[2]"=w667:u32, "LangsameHeizungen%[3]"=w666:u32, "LangsameHeizungen%[4]"=w665:u32, "LangsameHeizungen%[5]"=w664:u32)
        n62 = for {
          N: 1 -> [_]
          tunnel: w672 -> [w762]
          tunnel: [w762] -> w680
          tunnel: w669 -> [w761]
          n63 = call "Warten21"("Count(mSec)"=w761) -> ()  [unwired: 1 out]
        }
        n64 = for {
          N: 1 -> [_]
          tunnel: w672 -> [w739]
          tunnel: [w739] -> w677
          tunnel: w668 -> [w738]
          n65 = call "Warten24"("Count(mSec)"=w738) -> ()  [unwired: 1 out]
        }
        n66 = for {
          N: 1 -> [_]
          tunnel: w672 -> [w716]
          tunnel: [w716] -> w674
          tunnel: w667 -> [w715]
          n67 = call "Warten30"("Count(mSec)"=w715) -> ()  [unwired: 1 out]
        }
        n68 = for {
          N: 1 -> [_]
          tunnel: w672 -> [w808]
          tunnel: [w808] -> w686
          tunnel: w666 -> [w807]
          n69 = call "Warten15"("Count(mSec)"=w807) -> ()  [unwired: 1 out]
        }
        n70 = for {
          N: 1 -> [_]
          tunnel: w672 -> [w785]
          tunnel: [w785] -> w683
          tunnel: w665 -> [w784]
          n71 = call "Warten18"("Count(mSec)"=w784) -> ()  [unwired: 1 out]
        }
        n72 = for {
          N: 1 -> [_]
          tunnel: w672 -> [w831]
          tunnel: [w831] -> w689
          tunnel: w664 -> [w830]
          n73 = call "Warten12"("Count(mSec)"=w830) -> ()  [unwired: 1 out]
        }
        n74 = call "Warten9"("Count(mSec)"=u32 100) -> ()  [unwired: 1 out]
        n75 = xnode "Read/Write Control"("FPGA VI Reference In"=w680, "on/off Bronkhorst I Heater"=FALSE ("on/off T-Line Heater")) -> ()  [unwired: 1 in, 2 out]
        n76 = xnode "Read/Write Control"("FPGA VI Reference In"=w677, "on/off Main-Col I Heater"=FALSE ("on/off T-Line Heater")) -> ()  [unwired: 1 in, 2 out]
        n77 = xnode "Read/Write Control"("FPGA VI Reference In"=w674, "on/off Main-Col II Heater"=FALSE ("on/off T-Line Heater")) -> ()  [unwired: 1 in, 2 out]
        n78 = xnode "Read/Write Control"("FPGA VI Reference In"=w686, "on/off Bronkhorst II Heater"=FALSE ("on/off T-Line Heater")) -> ()  [unwired: 1 in, 2 out]
        n79 = xnode "Read/Write Control"("FPGA VI Reference In"=w683, "on/off Oven Heater"=FALSE ("on/off T-Line Heater")) -> ()  [unwired: 1 in, 2 out]
        n80 = xnode "Read/Write Control"("FPGA VI Reference In"=w689, "on/off T-Line Heater"=FALSE) -> ()  [unwired: 1 in, 2 out]
        n81 = global read "gvbooleschRT.vi" "global stop RT"() -> (w692:bool)
      }
      n82 = while {
        tunnel: w342 -> [w1222]
        shift-right: [w1217] -> _
        shift-left: w335 -> [w1211]
        shift-right: [w1216] -> _
        shift-left: w335 -> [w1209]
        shift-right: [w1214] -> _
        shift-left: w335 -> [w1215]
        shift-right: [w1212] -> _
        shift-left: w335 -> [w1213]
        shift-right: [w1218] -> _
        shift-left: _ -> [w1219]
        shift-right: ["dargestellte Größe 1"] -> _
        shift-left: _ -> [w1199]
        shift-right: ["Zeitachse1"] -> _
        shift-left: _ -> [w1201]
        shift-right: [w1185] -> _
        shift-left: w335 -> [w1193]
        shift-right: [w1186] -> _
        shift-left: w335 -> [w1192]
        shift-right: [w1191] -> _
        shift-left: w335 -> [w1189]
        shift-right: [w1190] -> _
        shift-left: w335 -> [w1188]
        shift-right: [w1178] -> _
        shift-left: _ -> [w1179]
        shift-right: ["Zeitachse2"] -> _
        shift-left: _ -> [w1177]
        shift-right: ["dargestellte Größe 2"] -> _
        shift-left: _ -> [w1175]
        stop <- w1226 stop-if-true
        n83 = local read "Big Ben, Methodenzeit, Zykluszeit0, Zykluszeit1, Zykluszeit2A, Zykluszeit2B"() -> (w1184:dbl[])
        n84 = local read "Zyklusnummern 0, 1, 2A, 2B"() -> (w1180:i32[])
        n85 = local read "Zyklnum1ges"() -> (w1196:i32)
        n86 = local read "Mod1Mod2Mod3/AITrapsMachs1Hz"() -> (w1198:dbl[])
        n87 = Index Array(array=w1180, index="Zeitachse1") -> (element=w1218:i32)
        n88 = To Double Precision Float(number=w1196) -> (double precision float=w1195:dbl)
        n89 = local read "MWHorst"() -> (w1197:dbl[])
        n90 = Index Array(array=w1180, index="Zeitachse2") -> (element=w1178:i32)
        n91 = Not Equal?(x=w1219, y=w1218) -> (x != y?=w1207:bool)
        n92 = Not Equal?(x="Zeitachse1", y=w1201) -> (x != y?=w1205:bool)
        n93 = To Double Precision Float(number=w1180) -> (double precision float=w1194:dbl[])
        n94 = local read "aktuelle TDMS-Datei"() -> (w1223:refnum<k34>)
        n95 = Not Equal?(x=w1179, y=w1178) -> (x != y?=w1173:bool)
        n96 = Not Equal?(x=w1177, y="Zeitachse2") -> (x != y?=w1172:bool)
        n97 = Not Equal?(x=w1175, y="dargestellte Größe 2") -> (x != y?=w1170:bool)
        n98 = Or(x=w1173, y=w1172) -> (x .or. y?=w1171:bool)
        n99 = Or(x=w1171, y=w1170) -> (x .or. y?=w1169:bool)
        n100 = Not Equal?(x="dargestellte Größe 1", y=w1199) -> (x != y?=w1204:bool)
        n101 = Or(x=w1207, y=w1205) -> (x .or. y?=w1206:bool)
        n102 = Build Array (concatenate)(w1195, w1194, w1184, w1198, w1197) -> (w1221:dbl[])
        n103 = Build Array (concatenate)(w1198, w1197) -> (w1183:dbl[])
        n104 = Index Array(array=w1184, index="Zeitachse2") -> (element=w1181:dbl)
        n105 = Index Array(array=w1183, index="dargestellte Größe 2") -> (element=w1182:dbl)
        n106 = Or(x=w1206, y=w1204) -> (x .or. y?=w1203:bool)
        n107 = TDMS Write(0:w1223, 1:enum16{"decimated", "interleaved"}."interleaved" ("Daten-Layout (0:dezimiert)"), 7:w1222, 9:w1221) -> ()  [unwired: 2 in, 4 out]
        n108 = Index Array(array=w1184, index="Zeitachse1") -> (element=w1210:dbl)
        n109 = Index Array(array=w1183, index="dargestellte Größe 1") -> (element=w1208:dbl)
        n110 = case shown="True" w1203 {
          tunnel: w1211 -> [w1247 w1251]
          tunnel: [w1245 w1255] -> w1217
          tunnel: [w1242 w1252] -> w1216
          tunnel: w1215 -> [w1249 _]
          tunnel: [w1249 w1251] -> w1214
          tunnel: w1213 -> [w1248 _]
          tunnel: [w1248 w1250] -> w1212
          tunnel: w1210 -> [w1246 w1256]
          tunnel: w1209 -> [w1244 w1250]
          tunnel: w1208 -> [w1243 w1253]
          frame False {
            n111 = Build Array (concatenate)(w1247, w1246) -> (w1245:dbl[])
            n112 = Build Array (concatenate)(w1244, w1243) -> (w1242:dbl[])
          }
          frame True {
            w1254 = dbl[] []
            n113 = Build Array (concatenate)(w1254, w1256) -> (w1255:dbl[])
            n114 = Build Array (concatenate)(w1254, w1253) -> (w1252:dbl[])
          }
        }
        n115 = case shown="True" w1169 {
          tunnel: w1193 -> [w1232 w1236]
          tunnel: [w1230 w1240] -> w1185
          tunnel: [w1227 w1237] -> w1186
          tunnel: w1189 -> [w1234 _]
          tunnel: [w1234 w1236] -> w1191
          tunnel: w1188 -> [w1233 _]
          tunnel: [w1233 w1235] -> w1190
          tunnel: w1181 -> [w1231 w1241]
          tunnel: w1192 -> [w1229 w1235]
          tunnel: w1182 -> [w1228 w1238]
          frame False {
            n116 = Build Array (concatenate)(w1232, w1231) -> (w1230:dbl[])
            n117 = Build Array (concatenate)(w1229, w1228) -> (w1227:dbl[])
          }
          frame True {
            w1239 = dbl[] []
            n118 = Build Array (concatenate)(w1239, w1241) -> (w1240:dbl[])
            n119 = Build Array (concatenate)(w1239, w1238) -> (w1237:dbl[])
          }
        }
        n120 = call "Warten6"("Count(mSec)"=u32 1000) -> ()  [unwired: 1 out]
        n121 = global read "gvbooleschRT.vi" "global stop RT"() -> (w1226:bool)
        n122 = Bundle(w1217, w1216) -> (→"Anzeige1":cluster{dbl[], dbl[]})  [unwired: 1 in]
        n123 = Bundle(w1185, w1186) -> (→"Anzeige2":cluster{dbl[], dbl[]})  [unwired: 1 in]
      }
      n124 = local read "PIDs für \"träge\" Heizungen"() -> (w346:T1)
      n125 = Add Array Elements(numeric array=w344) -> (sum=w343:i32)
      n126 = Compound Arithmetic op=ADD(w343, 8 ("Wert"), w348, w353) -> (w352:i32)
      n127 = for {
        N: w352 -> [_]
        tunnel: [FALSE] -> w355 mode=indexing
        tunnel: [0.0] -> w349 mode=indexing
      }
      n128 = Array To Cluster(array=w346) -> (cluster=w347:T17)
      n129 = while "\"langsame\" Regelungen" {
        tunnel: w364 -> [w902]
        tunnel: w347 -> [w910]
        stop <- w913 stop-if-true
        w911 = cluster{"output high":dbl, "output low":dbl} {"output high"=100.0, "output low"=0.0} ("output range")
        n130 = local read "Mod1/AI"() -> (w903:dbl[])
        n131 = call "Warten29"("Count(mSec)"=u32 100) -> ()  [unwired: 1 out]
        n132 = for {
          tunnel: w903 -> [w916]
          tunnel: w902 -> [w915] mode=indexing
          tunnel: [w914] -> w901 mode=indexing
          n133 = Index Array(array=w916, index=w915) -> (element=w914:dbl)
        }
        n134 = Array To Cluster(array="LangsameHeizungenSP") -> (cluster=w892:T18)
        n135 = Array To Cluster(array=w901) -> (cluster=w900:T19)
        n136 = Unbundle "Horst1\nMainCol1\nMainCol2\nHorst2\nOven\nT-line"(w892) -> ("LangsameHeizungenSP[0]"=w891:dbl, "LangsameHeizungenSP[1]"=w890:dbl, "LangsameHeizungenSP[2]"=w889:dbl, "LangsameHeizungenSP[3]"=w888:dbl, "LangsameHeizungenSP[4]"=w887:dbl, "LangsameHeizungenSP[5]"=w886:dbl)
        n137 = Unbundle "Horst1\nMainCol1\nMainCol2\nHorst2\nOven\nT-Line"(w900) -> ("[0]"=w899:dbl, "[1]"=w898:dbl, "[2]"=w897:dbl, "[3]"=w896:dbl, "[4]"=w895:dbl, "[5]"=w894:dbl)
        n138 = Unbundle "Horst1\nMainCol1\nMainCol2\nHorst2\nOven\nT-Line"(w910) -> ("PIDs für \"träge\" Heizungen[0]"=w909:T20, "PIDs für \"träge\" Heizungen[1]"=w908:T20, "PIDs für \"träge\" Heizungen[2]"=w907:T20, "PIDs für \"träge\" Heizungen[3]"=w906:T20, "PIDs für \"träge\" Heizungen[4]"=w905:T20, "PIDs für \"träge\" Heizungen[5]"=w904:T20)
        n139 = call-poly <vilib>:"PID.vi"("output range"=w911, "PID gains"=w908, "process variable"=w898, "setpoint"=w890) -> ("output"=w884:dbl)  [unwired: 6 in, 1 out]
        n140 = call-poly <vilib>:"PID.vi"("output range"=w911, "PID gains"=w907, "process variable"=w897, "setpoint"=w889) -> ("output"=w883:dbl)  [unwired: 6 in, 1 out]
        n141 = call-poly <vilib>:"PID.vi"("output range"=w911, "PID gains"=w909, "process variable"=w899, "setpoint"=w891) -> ("output"=w885:dbl)  [unwired: 6 in, 1 out]
        n142 = call-poly <vilib>:"PID.vi"("output range"=w911, "PID gains"=w906, "process variable"=w896, "setpoint"=w888) -> ("output"=w882:dbl)  [unwired: 6 in, 1 out]
        n143 = call-poly <vilib>:"PID.vi"("output range"=w911, "PID gains"=w904, "process variable"=w894, "setpoint"=w886) -> ("output"=w880:dbl)  [unwired: 6 in, 1 out]
        n144 = call-poly <vilib>:"PID.vi"("output range"=w911, "PID gains"=w905, "process variable"=w895, "setpoint"=w887) -> ("output"=w881:dbl)  [unwired: 6 in, 1 out]
        n145 = Build Array(w885, w884, w883, w882, w881, w880) -> (w879:dbl[])
        n146 = To Unsigned Long Integer(number=w879) -> (unsigned 32bit integer=w878:u32[])
        n147 = local write "LangsameHeizungen%"(w878) -> ()
        n148 = global read "gvbooleschRT.vi" "global stop RT"() -> (w913:bool)
      }
      n149 = Index Array(array=w370, index (col)=2 ("Deaktivierter Index (Spalte)")) -> (element=w392:dbl[])  [unwired: 1 in]
      n150 = Index Array(array=w370, index (col)=1 ("Deaktivierter Index (Spalte)")) -> (element=w390:dbl[])  [unwired: 1 in]
      n151 = Index Array(array=w370, index (col)=0 ("Deaktivierter Index (Spalte)")) -> (element=w388:dbl[])  [unwired: 1 in]
      n152 = Index Array(array=w369, index (col)=2 ("Deaktivierter Index (Spalte)")) -> (element=w384:dbl[])  [unwired: 1 in]
      n153 = Index Array(array=w369, index (col)=1 ("Deaktivierter Index (Spalte)")) -> (element=w383:dbl[])  [unwired: 1 in]
      n154 = Index Array(array=w369, index (col)=0 ("Deaktivierter Index (Spalte)")) -> (element=w382:dbl[])  [unwired: 1 in]
      n155 = Index Array(array=w368, index (col)=2 ("Deaktivierter Index (Spalte)")) -> (element=w378:dbl[])  [unwired: 1 in]
      n156 = Index Array(array=w368, index (col)=1 ("Deaktivierter Index (Spalte)")) -> (element=w377:dbl[])  [unwired: 1 in]
      n157 = Index Array(array=w368, index (col)=0 ("Deaktivierter Index (Spalte)")) -> (element=w376:dbl[])  [unwired: 1 in]
      n158 = Index Array(array=w360, index (col)=2 ("Deaktivierter Index (Spalte)")) -> (element=w359:dbl[])  [unwired: 1 in]
      n159 = Index Array(array=w360, index (col)=1 ("Deaktivierter Index (Spalte)")) -> (element=w358:dbl[])  [unwired: 1 in]
      n160 = Index Array(array=w360, index (col)=0 ("Deaktivierter Index (Spalte)")) -> (element=w357:dbl[])  [unwired: 1 in]
      n161 = while {
        stop <- w933 stop-if-true
        w918 = 10.0
        n162 = call "Warten27"("Count(mSec)"=u32 1000) -> ()  [unwired: 1 out]
        n163 = local read "Traps/Machs"() -> (w920:dbl[])
        n164 = local read "Mod1/AI"() -> (w931:dbl[])
        n165 = local read "Mod2/AI"() -> (w930:dbl[])
        n166 = local read "Mod3/AI"() -> (w929:dbl[])
        n167 = for {
          N: 9 -> [_]
          shift-right: [w940] -> w927
          shift-left: w931 -> [w941]
          shift-right: [w938] -> w926
          shift-left: w930 -> [w939]
          shift-right: [w936] -> w925
          shift-left: w929 -> [w937]
          shift-right: [w934] -> w919
          shift-left: w920 -> [w935]
          n168 = flat-sequence {
            tunnel: w941 -> [w954]
            tunnel: [w952] -> w940
            tunnel: w939 -> [w951]
            tunnel: [w949] -> w938
            tunnel: w937 -> [w948]
            tunnel: [w946] -> w936
            tunnel: w935 -> [w944]
            tunnel: [w943] -> w934
            frame #0 {
              n169 = call "Warten28"("Count(mSec)"=u32 100) -> ()  [unwired: 1 out]
            }
            frame #1 {
              n170 = local read "Traps/Machs"() -> (w945:dbl[])
              n171 = local read "Mod1/AI"() -> (w953:dbl[])
              n172 = local read "Mod2/AI"() -> (w950:dbl[])
              n173 = local read "Mod3/AI"() -> (w947:dbl[])
              n174 = Add(x=w954, y=w953) -> (x+y=w952:dbl[])
              n175 = Add(x=w951, y=w950) -> (x+y=w949:dbl[])
              n176 = Add(x=w948, y=w947) -> (x+y=w946:dbl[])
              n177 = Add(x=w945, y=w944) -> (x+y=w943:dbl[])
            }
          }
        }
        n178 = Divide(x=w927, y=w918) -> (x/y=w924:dbl[])
        n179 = Divide(x=w926, y=w918) -> (x/y=w923:dbl[])
        n180 = Divide(x=w925, y=w918) -> (x/y=w922:dbl[])
        n181 = Divide(x=w919, y=w918) -> (x/y=w917:dbl[])
        n182 = Build Array (concatenate)(w924, w923, w922, w917) -> (→"Mod1Mod2Mod3/AITrapsMachs1Hz":dbl[])
        n183 = global read "gvbooleschRT.vi" "global stop RT"() -> (w933:bool)
      }
      n184 = while {
        tunnel: w355 -> [w1296]
        tunnel: w344 -> [w1275]
        tunnel: w353 -> [w1280]
        tunnel: w348 -> [w1282]
        tunnel: w350 -> [w1292]
        tunnel: w349 -> [w1290]
        tunnel: w343 -> [w1274]
        stop <- "global stop RT" stop-if-true
        w1268 = 2 ("Index")
        w1287 = 6 ("Index")
        n185 = local read "Zwangsbedingungen"() -> (w1278:dbl[][])
        n186 = local read "Mod1Mod2Mod3/AITrapsMachs1Hz"() -> (w1299:dbl[])
        n187 = call "Warten5"("Count(mSec)"=u32 1000) -> ()  [unwired: 1 out]
        n188 = local read "MWHorst"() -> (w1298:dbl[])
        n189 = Build Array (concatenate)(w1299, w1298) -> (w1297:dbl[])
        n190 = for {
          tunnel: w1297 -> [w1338]
          tunnel: w1278 -> [w1336] mode=indexing
          shift-right: [w1329] -> w1295
          shift-left: w1296 -> [w1335]
          shift-right: [w1330] -> w1289
          shift-left: w1290 -> [w1334]
          n191 = Index Array(array=w1336, index=0 ("Index")) -> (element=w1348:dbl)
          n192 = Index Array(array=w1336, index=1 ("Index")) -> (element=w1346:dbl)
          n193 = Index Array(array=w1336, index=2 ("Index")) -> (element=w1342:dbl)
          n194 = Index Array(array=w1336, index=3 ("Index")) -> (element=w1339:dbl)
          n195 = Index Array(array=w1336, index=4 ("Index")) -> (element=w1331:dbl)
          n196 = To Long Integer(number=w1348) -> (32bit integer=w1341:i32)
          n197 = To Long Integer(number=w1346) -> (32bit integer=w1345:i32)
          n198 = To Long Integer(number=w1339) -> (32bit integer=w1333:i32)
          n199 = Index Array(array=w1338, index=w1341) -> (element=w1344:dbl)
          n200 = case shown="0, Default" w1345 {
            tunnel: w1344 -> [w1361 w1363 w1367 w1370 w1373 w1376]
            tunnel: w1342 -> [w1360 w1364 w1366 w1369 w1372 w1375]
            tunnel: [w1359 w1362 w1365 w1368 w1371 w1374] -> w1332
            frame 0, Default {
              n201 = Less?(x=w1361, y=w1360) -> (x < y?=w1359:bool)
            }
            frame 1 {
              n202 = Less Or Equal?(x=w1363, y=w1364) -> (x <= y?=w1362:bool)
            }
            frame 2 {
              n203 = Equal?(x=w1367, y=w1366) -> (x = y?=w1365:bool)
            }
            frame 3 {
              n204 = Greater Or Equal?(x=w1370, y=w1369) -> (x >= y?=w1368:bool)
            }
            frame 4 {
              n205 = Greater?(x=w1373, y=w1372) -> (0:w1371:bool)
            }
            frame 5 {
              n206 = Not Equal?(x=w1376, y=w1375) -> (x != y?=w1374:bool)
            }
          }
          n207 = case shown="True" w1332 {
            tunnel: w1335 -> [w1351 w1358]
            tunnel: w1334 -> [w1350 w1357]
            tunnel: w1333 -> [_ w1356]
            tunnel: w1332 -> [_ w1355]
            tunnel: w1331 -> [_ w1354]
            tunnel: [w1350 w1353] -> w1330
            tunnel: [w1351 w1352] -> w1329
            frame False {
            }
            frame True {
              n208 = Replace Array Subset(array=w1358, new element=w1355, index=w1356) -> (w1352:bool[])
              n209 = Replace Array Subset(array=w1357, new element=w1354, index=w1356) -> (w1353:dbl[])
            }
          }
        }
        n210 = global write "gvbooleschRT.vi" "global stop RT"("global stop RT") -> ()
        n211 = Split 1D Array ("DIO")(array=w1289, index=w1274) -> (first subarray=w1288:dbl[], second subarray=w1286:dbl[])
        n212 = Split 1D Array "DIO"(array=w1295, index=w1274) -> (first subarray=w1261:bool[], second subarray=w1294:bool[])
        n213 = Split 1D Array(array=w1286, index=w1287) -> (first subarray=w1284:dbl[], second subarray=w1270:dbl[])
        n214 = Split 1D Array "FPGABoolesch"(array=w1294, index=w1287) -> (first subarray=→"ZwangsFPGABoolesch?":bool[], second subarray=w1272:bool[])
        n215 = Split 1D Array "Methodenübergreifend"(array=w1272, index=w1268) -> (first subarray=w1265:bool[], second subarray=w1271:bool[])
        n216 = Split 1D Array "LangsameHeizungen"(array=w1271, index=w1282) -> (first subarray=→"ZwangsLangsameH?":bool[], second subarray=w1293:bool[])
        n217 = Split 1D Array "BronkhorstSP"(array=w1293, index=w1280) -> (first subarray=w1291:bool[])  [unwired: 1 out]
        n218 = Split 1D Array(array=w1270, index=w1268) -> (first subarray=w1262:dbl[], second subarray=w1269:dbl[])
        n219 = Split 1D Array(array=w1269, index=w1282) -> (first subarray=w1277:dbl[], second subarray=w1281:dbl[])
        n220 = Split 1D Array(array=w1281, index=w1280) -> (first subarray=w1279:dbl[])  [unwired: 1 out]
        n221 = for {
          tunnel: [w1321] -> w1260 mode=indexing
          tunnel: w1275 -> [w1323] mode=indexing
          tunnel: [w1319] -> w1259 mode=indexing
          shift-right: [w1327] -> _
          shift-left: w1261 -> [w1328]
          shift-right: [w1325] -> _
          shift-left: w1288 -> [w1326]
          n222 = Split 1D Array(array=w1326, index=w1323) -> (first subarray=w1324:dbl[], second subarray=w1325:dbl[])
          n223 = Split 1D Array(array=w1328, index=w1323) -> (first subarray=w1322:bool[], second subarray=w1327:bool[])
          n224 = Greater Than 0?(x=w1324) -> (x > 0?=w1320:bool[])
          n225 = Bundle(w1322) -> (w1321:cluster{bool[]})  [unwired: 1 in]
          n226 = Bundle(w1320) -> (w1319:cluster{bool[]})  [unwired: 1 in]
        }
        "ZwangsDIO?" <- w1260
        "ZwangsDIO!" <- w1259
        n227 = for {
          tunnel: w1292 -> [w1315] mode=indexing
          shift-right: [w1317] -> _
          shift-left: w1291 -> [w1318]
          tunnel: [w1312] -> w1258 mode=indexing
          shift-right: [w1314] -> _
          shift-left: w1279 -> [w1316]
          tunnel: [w1310] -> w1257 mode=indexing
          n228 = Split 1D Array(array=w1318, index=w1315) -> (first subarray=w1313:bool[], second subarray=w1317:bool[])
          n229 = Split 1D Array(array=w1316, index=w1315) -> (first subarray=w1311:dbl[], second subarray=w1314:dbl[])
          n230 = Bundle(w1313) -> (w1312:cluster{bool[]})  [unwired: 1 in]
          n231 = Bundle(w1311) -> (w1310:cluster{dbl[]})  [unwired: 1 in]
        }
        "ZwangsHorst?" <- w1258
        "ZwangsHorst!" <- w1257
        n232 = Greater Than 0?(x=w1284) -> (x > 0?=→"ZwangsFPGABoolesch!":bool[])
        n233 = Index Array(array=w1265, index=0 ("Index")) -> (element=w1266:bool)
        n234 = Greater Than 0?(x=w1277) -> (x > 0?=→"ZwangsLangsameH!":bool[])
        n235 = Index Array(array=w1265, index=1 ("Index")) -> (element=w1263:bool)
        n236 = case shown="True" w1266 {
          tunnel: w1262 -> [_ w1308]
          frame False {
          }
          frame True {
            n237 = Index Array(array=w1308, index=0 ("Index")) -> (element=w1307:dbl)
            n238 = To Long Integer(number=w1307) -> (32bit integer=w1306:i32)
            n239 = local write "Methodennummer"(w1306) -> ()
          }
        }
        n240 = case shown="True" w1263 {
          tunnel: w1262 -> [_ w1305]
          frame False {
          }
          frame True {
            n241 = Index Array(array=w1305, index=1 ("Index")) -> (element=w1303:dbl)
            n242 = Greater Than 0?(x=w1303) -> (x > 0?=w1302:bool)
            n243 = local write "global stop RT"(w1302) -> ()
          }
        }
      }
      n244 = for {
        N: 64 -> [_]
        tunnel: [FALSE] -> w365 mode=indexing
      }
      n245 = while "AIMittelwerte" {
        tunnel: w367 -> [w1008]
        tunnel: w392 -> [w999]
        tunnel: w390 -> [w998]
        tunnel: w388 -> [w994]
        tunnel: w384 -> [w987]
        tunnel: w383 -> [w985]
        tunnel: w382 -> [w984]
        tunnel: w378 -> [w977]
        tunnel: w377 -> [w976]
        tunnel: w376 -> [w975]
        tunnel: w359 -> [w958]
        tunnel: w358 -> [w957]
        tunnel: w357 -> [w956]
        stop <- w1013 stop-if-true
        w964 = 10.0
        n246 = xnode "Read/Write Control"("FPGA VI Reference In"=w1008) -> ("Mod1/AI"=w1007:void[], "Mod2/AI"=w1006:void[], "Mod3/AI"=w1005:void[], "UWidr[V]Trap1"=w973, "UTemp[V]Trap1"=w972, "UWidr[V]Trap2"=w971, "UTemp[V]Trap2"=w970, "U[V]Mach1"=w969, "U[V]Mach2"=w968)  [unwired: 1 in, 2 out]
        n247 = call "Warten26"("Count(mSec)"=u32 100) -> ()  [unwired: 1 out]
        n248 = To Double Precision Float(number=w1007) -> (double precision float=w1004:dbl[])
        n249 = To Double Precision Float(number=w1006) -> (double precision float=w1003:dbl[])
        n250 = To Double Precision Float(number=w1005) -> (double precision float=w1002:dbl[])
        n251 = Build Array(w973, w972, w971, w970, w969, w968) -> (w967:void[])
        n252 = To Double Precision Float(number=w967) -> (double precision float=w966:dbl[])
        n253 = for {
          N: 9 -> [_]
          shift-right: [w1080] -> w1011
          shift-left: w1004 -> [w1083]
          shift-right: [w1079] -> w1010
          shift-left: w1003 -> [w1082]
          shift-right: [w1078] -> w1009
          shift-left: w1002 -> [w1081]
          tunnel: w1008 -> [w1077]
          shift-right: [w1075] -> w965
          shift-left: w966 -> [w1076]
          n254 = flat-sequence {
            tunnel: w1083 -> [w1101]
            tunnel: w1082 -> [w1100]
            tunnel: w1081 -> [w1099]
            tunnel: [w1098] -> w1080
            tunnel: [w1097] -> w1079
            tunnel: [w1096] -> w1078
            tunnel: w1077 -> [w1095]
            tunnel: w1076 -> [w1086]
            tunnel: [w1085] -> w1075
            frame #0 {
              n255 = call "Warten4"("Count(mSec)"=u32 10) -> ()  [unwired: 1 out]
            }
            frame #1 {
              n256 = xnode "Read/Write Control"("FPGA VI Reference In"=w1095) -> ("Mod1/AI"=w1105:void[], "Mod2/AI"=w1106:void[], "Mod3/AI"=w1107:void[], "UWidr[V]Trap1"=w1094, "UTemp[V]Trap1"=w1093, "UWidr[V]Trap2"=w1092, "UTemp[V]Trap2"=w1091, "U[V]Mach1"=w1090, "U[V]Mach2"=w1089)  [unwired: 1 in, 2 out]
              n257 = Build Array(w1094, w1093, w1092, w1091, w1090, w1089) -> (w1088:void[])
              n258 = To Double Precision Float(number=w1105) -> (double precision float=w1104:dbl[])
              n259 = To Double Precision Float(number=w1106) -> (double precision float=w1103:dbl[])
              n260 = To Double Precision Float(number=w1107) -> (double precision float=w1102:dbl[])
              n261 = To Double Precision Float(number=w1088) -> (double precision float=w1087:dbl[])
              n262 = Add(x=w1101, y=w1104) -> (x+y=w1098:dbl[])
              n263 = Add(x=w1100, y=w1103) -> (x+y=w1097:dbl[])
              n264 = Add(x=w1099, y=w1102) -> (x+y=w1096:dbl[])
              n265 = Add(x=w1086, y=w1087) -> (x+y=w1085:dbl[])
            }
          }
        }
        n266 = Divide(x=w965, y=w964) -> (x/y=w963:dbl[])
        n267 = Divide(x=w1011, y=w964) -> (x/y=w997:dbl[])
        n268 = Divide(x=w1010, y=w964) -> (x/y=w986:dbl[])
        n269 = Divide(x=w1009, y=w964) -> (x/y=w980:dbl[])
        n270 = Square(x=w963) -> (x^2=w962:dbl[])
        n271 = Multiply(x=w962, y=w958) -> (x*y=w961:dbl[])
        n272 = Multiply(x=w963, y=w957) -> (x*y=w960:dbl[])
        n273 = Multiply(x=w997, y=w998) -> (x*y=w995:dbl[])
        n274 = Multiply(x=w986, y=w985) -> (x*y=w989:dbl[])
        n275 = Multiply(x=w980, y=w976) -> (x*y=w978:dbl[])
        n276 = Square(x=w997) -> (x^2=w1000:dbl[])
        n277 = Square(x=w986) -> (x^2=w991:dbl[])
        n278 = Square(x=w980) -> (x^2=w981:dbl[])
        n279 = Add(x=w961, y=w960) -> (x+y=w959:dbl[])
        n280 = Multiply(x=w1000, y=w999) -> (x*y=w996:dbl[])
        n281 = Multiply(x=w991, y=w987) -> (x*y=w990:dbl[])
        n282 = Multiply(x=w981, y=w977) -> (x*y=w979:dbl[])
        n283 = Add(x=w959, y=w956) -> (x+y=→"Traps/Machs":dbl[])
        n284 = Add(x=w996, y=w995) -> (x+y=w993:dbl[])
        n285 = Add(x=w990, y=w989) -> (x+y=w988:dbl[])
        n286 = Add(x=w979, y=w978) -> (x+y=w982:dbl[])
        n287 = Add(x=w993, y=w994) -> (x+y=→"Mod1/AI":dbl[])
        n288 = Add(x=w988, y=w984) -> (x+y=→"Mod2/AI":dbl[])
        n289 = Add(x=w982, y=w975) -> (x+y=→"Mod3/AI":dbl[])
        n290 = global read "gvbooleschRT.vi" "global stop RT"() -> (w1013:bool)
      }
      n291 = while "Methoden- und Zyklussteuerung" {
        shift-right: [w1441] -> _
        shift-left: 0.0 -> [w1440]
        shift-right: [w1439] -> _
        shift-left: -1 -> [w1438]
        tunnel: w367 -> [w1428]
        tunnel: w356 -> [w1432]
        tunnel: w365 -> [w1431]
        tunnel: w351 -> [w1421]
        tunnel: w345 -> [w1420]
        i -> [w1444]
        stop <- w1445 stop-if-true
        w1422 = 0  # ZeileMach2
        w1423 = 0  # ZeileMach1
        w1424 = 0  # ZeileFPGAFixp
        w1425 = 0  # ZeileFPGAPID
        w1427 = 0  # ZeileFPGABoolesch
        w1430 = i32[] [0, 0, 0, 0]  # ZeilennummernHorst
        w1435 = i32[] [0, 0, 0, 0]  # ZeilennummernDIOs
        n292 = local read "Methodennummer"() -> (w1419:i32)
        n293 = Index Array(array=w1420, index=w1419) -> (element=w1418:T21)
        n294 = Unbundle(w1418) -> ("Zykluslängen [s]"=w1417:dbl[], "ZeitpktDIOsMod0"=w1387:dbl[], "ZeitpktDIOsMod1"=w1386:dbl[], "ZeitpktDIOsMod2A"=w1385:dbl[], "ZeitpktDIOsMod2B"=w1384:dbl[], "DIOsSPMod0"=w1392:bool[][], "DIOsSPMod1"=w1391:bool[][], "DIOsSPMod2A"=w1390:bool[][], "DIOsSPMod2B"=w1389:bool[][], "Mod0HorstZeitpkt"=w1397:dbl[], "Mod1HorstZeitpkt"=w1396:dbl[], "Mod2AHorstZeitpkt"=w1395:dbl[], "Mod2BHorstZeitpkt"=w1394:dbl[], "HorstSPMod0"=w1402:dbl[][], "HorstSPMod1"=w1401:dbl[][], "HorstSPMod2A"=w1400:dbl[][], "HorstSPMod2B"=w1399:dbl[][], "LangsameHeizungenSP"=w1416:dbl[], "LHHeizen?"=w1415:bool[], "ZPktFPGABoolesch"=w1413:dbl[], "FPGABoolesch"=w1412:bool[][], "ZeitpktFPGAPID"=w1411:dbl[], "FPGAPID"=w1410:T22, "ZeitpktFPGAFixp"=w1409:dbl[], "FPGAFixp"=w1408:fxp<+/-,16,4>[][], "ZeitpktMach1"=w1407:dbl[], "TempMach1"=w1406:dbl[], "ZeitpktMach2"=w1405:dbl[], "TempMach2"=w1404:dbl[], "PIDs für \"träge\" Heizungen"=→"PIDs für \"träge\" Heizungen":T1, "Zwangsbedingungen"=→"Zwangsbedingungen":dbl[][], "Text0 MS-Datei"=w1382:string, "Info"=w1381:string, "wie wird gespeichert?"=w1380:u16, "Speicherlänge"=w1379:string, "Dateien fürs MS schicken?"=w1378:bool, "Pfad MS-Datei CRIO"=w1377:path)
        n295 = local write "LangsameHeizungenSP"(w1416) -> ()
        n296 = local write "Text0 MS-Datei"(w1382) -> ()
        n297 = local write "wie wird gespeichert?"(w1380) -> ()
        n298 = Build Cluster Array(w1397, w1396, w1395, w1394) -> (w1393:cluster{"Mod2BHorstZeitpkt":dbl[]}[])
        n299 = Build Cluster Array(w1402, w1401, w1400, w1399) -> (w1398:cluster{"HorstSPMod2B":dbl[][]}[])
        n300 = Build Cluster Array(w1392, w1391, w1390, w1389) -> (w1388:cluster{"DIOsSPMod2B":bool[][]}[])
        n301 = local write "Speicherlänge"(w1379) -> ()
        n302 = local write "Info"(w1381) -> ()
        n303 = local write "Pfad MS-Datei CRIO"(w1377) -> ()
        n304 = local write "Dateien fürs MS schicken?"(w1378) -> ()
        n305 = Build Cluster Array(w1387, w1386, w1385, w1384) -> (w1383:cluster{"ZeitpktDIOsMod2B":dbl[]}[])
        n306 = Add(x=w1438, y=1) -> (x+y=w1436:i32)
        n307 = local read "Zyklusnummern 0, 1, 2A, 2B"() -> (w1434:i32[])
        n308 = local read "ZwangsFPGABoolesch?"() -> (w1426:bool[])
        n309 = local read "ZwangsHorst?"() -> (w1429:cluster{bool[]}[])
        n310 = local read "ZwangsDIO?"() -> (w1433:cluster{bool[]}[])
        n311 = while "ZyklusSteuerung" {
          shift-right: [w1599] -> _
          shift-left: w1434 -> [w1598]
          shift-right: [w1591] -> _
          shift-left: w1435 -> [w1596]
          tunnel: w1383 -> [w1594]
          shift-right: [w1449] -> _
          shift-left: w1433 -> [w1450]
          tunnel: w1388 -> [w1447]
          tunnel: w1432 -> [w1585]
          tunnel: w1431 -> [w1584]
          tunnel: w1428 -> [w1506]
          tunnel: w1393 -> [w1582]
          shift-right: [w1579] -> _
          shift-left: w1430 -> [w1583]
          shift-right: [w1452] -> _
          shift-left: w1429 -> [w1453]
          tunnel: w1398 -> [w1456]
          shift-right: [w1566] -> _
          shift-left: w1427 -> [w1572]
          tunnel: w1413 -> [w1573]
          tunnel: w1412 -> [w1559]
          shift-right: [w1560] -> _
          shift-left: w1426 -> [w1564]
          tunnel: w1411 -> [w1557]
          shift-right: [w1553] -> _
          shift-left: w1425 -> [w1558]
          tunnel: w1410 -> [w1551]
          shift-right: [w1544] -> _
          shift-left: w1424 -> [w1549]
          tunnel: w1409 -> [w1548]
          tunnel: w1408 -> [w1542]
          shift-right: [w1529] -> _
          shift-left: w1423 -> [w1540]
          tunnel: w1407 -> [w1538]
          tunnel: w1406 -> [w1537]
          shift-right: [w1472] -> _
          shift-left: w1422 -> [w1474]
          tunnel: w1405 -> [w1471]
          tunnel: w1404 -> [w1470]
          tunnel: w1421 -> [_]
          tunnel: w1415 -> [w1467]
          stop <- w1602 stop-if-true
          w1478 = 6.0782 ("y")
          w1511 = 6.0782 ("y")
          n312 = local read "ZwangsHorst?"() -> (w1452:cluster{bool[]}[])
          n313 = local read "ZwangsFPGABoolesch?"() -> (w1560:bool[])
          n314 = local read "Zyklusnummern 0, 1, 2A, 2B"() -> (w1599:i32[])
          n315 = local read "ZwangsDIO?"() -> (w1449:cluster{bool[]}[])
          n316 = Not Equal?(x=w1560, y=w1564) -> (x != y?=w1563:bool)
          n317 = Not Equal?(x=w1450, y=w1449) -> (x != y?=w1448:bool)
          n318 = Equal?(x=w1599, y=w1598) -> (x = y?=w1597:bool[])
          n319 = local read "ZwangsLangsameH?"() -> (w1465:bool[])
          n320 = Not Equal?(x=w1452, y=w1453) -> (x != y?=w1451:bool)
          n321 = local read "ZwangsLangsameH!"() -> (w1464:bool[])
          n322 = Boolean To (0,1)(Boolean=w1597) -> (0, 1=w1595:i16[])
          n323 = To Long Integer(number=w1595) -> (32bit integer=w1575:i32[])
          n324 = Multiply(x=w1575, y=w1583) -> (x*y=w1454:i32[])
          n325 = Index Array(array=w1575, index=1 ("Index")) -> (element=w1473:i32)
          n326 = Multiply(x=w1473, y=w1540) -> (x*y=w1530:i32)
          n327 = Multiply(x=w1473, y=w1549) -> (x*y=w1543:i32)
          n328 = Multiply(x=w1473, y=w1474) -> (x*y=w1498:i32)
          n329 = Add(x=1 ("y"), y=w1530) -> (x+y=w1536:i32)
          n330 = Index Array(array=w1548, index=w1543) -> (element=w1547:dbl)
          n331 = Add(x=1 ("y"), y=w1498) -> (x+y=w1504:i32)
          n332 = Multiply(x=w1473, y=w1558) -> (x*y=w1550:i32)
          n333 = Index Array(array=w1538, index=w1530) -> (element=w1528:dbl)
          n334 = Index Array(array=w1538, index=w1536) -> (element=w1534:dbl)
          n335 = Multiply(x=w1473, y=w1572) -> (x*y=w1561:i32)
          n336 = Index Array(array=w1573, index=w1561) -> (element=w1569:dbl)
          n337 = Index Array(array=w1537, index=w1530) -> (element=w1522:dbl)
          n338 = Index Array(array=w1537, index=w1536) -> (element=w1535:dbl)
          n339 = Index Array(array=w1471, index=w1498) -> (element=w1497:dbl)
          n340 = Index Array(array=w1471, index=w1504) -> (element=w1502:dbl)
          n341 = Index Array(array=w1470, index=w1498) -> (element=w1491:dbl)
          n342 = Index Array(array=w1470, index=w1504) -> (element=w1503:dbl)
          n343 = Index Array(array=w1557, index=w1550) -> (element=w1556:dbl)
          n344 = Subtract(x=w1534, y=w1528) -> (x-y=w1526:dbl)
          n345 = Subtract(x=w1535, y=w1522) -> (x-y=w1524:dbl)
          n346 = Subtract(x=w1502, y=w1497) -> (x-y=w1495:dbl)
          n347 = Subtract(x=w1503, y=w1491) -> (x-y=w1493:dbl)
          n348 = Multiply(x=w1575, y=w1596) -> (x*y=w1458:i32[])
          n349 = Not(x=w1465) -> (.not. x?=w1466:bool[])
          n350 = local read "Zykluszeiten 0, 1, 2A, 2B"() -> (w1571:dbl[])
          n351 = Index Array(array=w1571, index=1 ("Index")) -> (element=w1469:dbl)
          n352 = Greater Or Equal?(x=w1469, y=w1547) -> (x >= y?=w1541:bool)
          n353 = Boolean To (0,1)(Boolean=w1541) -> (0, 1=w1546:i16)
          n354 = Greater Or Equal?(x=w1469, y=w1534) -> (x >= y?=w1533:bool)
          n355 = To Long Integer(number=w1546) -> (32bit integer=w1545:i32)
          n356 = Greater Or Equal?(x=w1469, y=w1502) -> (x >= y?=w1501:bool)
          n357 = Greater Or Equal?(x=w1469, y=w1556) -> (x >= y?=w1552:bool)
          n358 = Subtract(x=w1469, y=w1528) -> (x-y=w1527:dbl)
          n359 = Greater Or Equal?(x=w1469, y=w1569) -> (x >= y?=w1565:bool)
          n360 = Boolean To (0,1)(Boolean=w1533) -> (0, 1=w1532:i16)
          n361 = Subtract(x=w1469, y=w1497) -> (x-y=w1496:dbl)
          n362 = Add(x=w1543, y=w1545) -> (x+y=w1544:i32)
          n363 = Boolean To (0,1)(Boolean=w1501) -> (0, 1=w1500:i16)
          n364 = Boolean To (0,1)(Boolean=w1552) -> (0, 1=w1555:i16)
          n365 = Divide(x=w1527, y=w1526) -> (x/y=w1525:dbl)
          n366 = Boolean To (0,1)(Boolean=w1565) -> (0, 1=w1568:i16)
          n367 = To Long Integer(number=w1532) -> (32bit integer=w1531:i32)
          n368 = Or(x=w1565, y=w1563) -> (x .or. y?=w1562:bool)
          n369 = for {
            tunnel: w1454 -> [w1841] mode=indexing
            tunnel: w1571 -> [w1840] mode=indexing
            tunnel: w1582 -> [w1837] mode=indexing
            tunnel: [w1838] -> w1455 mode=indexing
            n370 = Unbundle(w1837) -> ("Mod2BHorstZeitpkt"=w1836:dbl[])
            n371 = Index Array(array=w1836, index=w1841) -> (element=w1839:dbl)
            n372 = Greater Or Equal?(x=w1840, y=w1839) -> (x >= y?=w1838:bool)
          }
          n373 = Divide(x=w1496, y=w1495) -> (x/y=w1494:dbl)
          n374 = Multiply(x=w1525, y=w1524) -> (x*y=w1523:dbl)
          n375 = To Long Integer(number=w1555) -> (32bit integer=w1554:i32)
          n376 = To Long Integer(number=w1500) -> (32bit integer=w1499:i32)
          n377 = And(x=w1465, y=w1464) -> (x .and. y?=w1462:bool[])
          n378 = for {
            tunnel: w1458 -> [w1914] mode=indexing
            tunnel: w1571 -> [w1913] mode=indexing
            tunnel: [w1912] -> w1446 mode=indexing
            tunnel: w1594 -> [w1910] mode=indexing
            n379 = Unbundle(w1910) -> ("ZeitpktDIOsMod2B"=w1909:dbl[])
            n380 = Index Array(array=w1909, index=w1914) -> (element=w1911:dbl)
            n381 = Greater Or Equal?(x=w1913, y=w1911) -> (x >= y?=w1912:bool)
          }
          n382 = To Long Integer(number=w1568) -> (32bit integer=w1567:i32)
          n383 = Add(x=w1523, y=w1522) -> (x+y=w1508:dbl)
          n384 = Multiply(x=w1494, y=w1493) -> (x*y=w1492:dbl)
          n385 = And(x=w1466, y=w1467) -> (x .and. y?=w1463:bool[])
          n386 = Add(x=w1530, y=w1531) -> (x+y=w1529:i32)
          n387 = Add(x=w1550, y=w1554) -> (x+y=w1553:i32)
          n388 = case shown="True" w1541 {
            tunnel: w1543 -> [_ w1659]
            tunnel: w1542 -> [_ w1671]
            tunnel: w1506 -> [_ w1661]
            frame False {
            }
            frame True {
              n389 = Index Array(array=w1671, index (row)=w1659) -> (element=w1660:fxp<+/-,16,4>[])  [unwired: 1 in]
              n390 = Array To Cluster(array=w1660) -> (cluster=w1670:T23)
              n391 = Unbundle(w1670) -> ("FPGAFixp[0]"=w1669:fxp<+/-,16,4>, "FPGAFixp[1]"=w1668:fxp<+/-,16,4>, "FPGAFixp[2]"=w1667:fxp<+/-,16,4>, "FPGAFixp[3]"=w1666:fxp<+/-,16,4>, "FPGAFixp[4]"=w1665:fxp<+/-,16,4>, "FPGAFixp[5]"=w1664:fxp<+/-,16,4>, "FPGAFixp[6]"=w1663:fxp<+/-,16,4>, "FPGAFixp[7]"=w1662:fxp<+/-,16,4>)
              n392 = xnode "Read/Write Control"("FPGA VI Reference In"=w1661, "UTempSPTrap1"=w1669, "UTempMaxTrap1"=w1668, "UWidrMaxTrap1"=w1667, "UTempSPTrap2"=w1666, "UTempMaxTrap2"=w1665, "UWidrMaxTrap2"=w1664, "Umax[V]Mach1"=w1663, "Umax[V]Mach2"=w1662) -> ()  [unwired: 1 in, 2 out]
            }
          }
          n393 = Add(x=w1492, y=w1491) -> (x+y=w1475:dbl)
          n394 = Add(x=w1498, y=w1499) -> (x+y=w1472:i32)
          n395 = Add(x=w1561, y=w1567) -> (x+y=w1566:i32)
          n396 = Or(x=w1463, y=w1462) -> (x .or. y?=w1461:bool[])
          n397 = local write "Heizen?LH"(w1461) -> ()
          n398 = case shown="True" w1552 {
            tunnel: w1506 -> [_ w1736]
            tunnel: w1551 -> [_ w1735]
            tunnel: w1550 -> [_ w1728]
            frame False {
            }
            frame True {
              n399 = Index Array(array=w1735, index (row)=w1728) -> (element=w1734:T24)  [unwired: 1 in]
              n400 = Array To Cluster(array=w1734) -> (cluster=w1733:T25)
              n401 = Unbundle(w1733) -> ("FPGAPID[0]"=w1732:T26, "FPGAPID[1]"=w1731:T26, "FPGAPID[2]"=w1730:T26, "FPGAPID[3]"=w1729:T26)
              n402 = xnode "Read/Write Control"("FPGA VI Reference In"=w1736, "PIDTrap1"=w1732, "PIDTrap2"=w1731, "PIDMach1"=w1730, "PIDMach2"=w1729) -> ()  [unwired: 1 in, 2 out]
            }
          }
          n403 = case shown="True" w1562 {
            tunnel: w1561 -> [_ w1773]
            tunnel: w1560 -> [_ w1784]
            tunnel: w1559 -> [_ w1789]
            tunnel: w1506 -> [_ w1781]
            frame False {
            }
            frame True {
              n404 = local read "ZwangsFPGABoolesch!"() -> (w1785:bool[])
              n405 = Index Array(array=w1789, index (row)=w1773) -> (element=w1787:bool[])  [unwired: 1 in]
              n406 = Not(x=w1784) -> (.not. x?=w1788:bool[])
              n407 = And(x=w1787, y=w1788) -> (x .and. y?=w1786:bool[])
              n408 = And(x=w1784, y=w1785) -> (x .and. y?=w1783:bool[])
              n409 = Or(x=w1786, y=w1783) -> (x .or. y?=w1782:bool[])
              n410 = Array To Cluster(array=w1782) -> (cluster=w1780:T27)
              n411 = Unbundle(w1780) -> ("[0]"=w1779:bool, "[1]"=w1778:bool, "[2]"=w1777:bool, "[3]"=w1776:bool, "[4]"=w1775:bool, "[5]"=w1774:bool)
              n412 = xnode "Read/Write Control"("FPGA VI Reference In"=w1781, "ServoTrap1kalt"=w1779, "ServoTrap2kalt"=w1778, "Heizen?Trap1"=w1777, "Heizen?Trap2"=w1776, "Heizen?Mach1"=w1775, "Heizen?Mach2"=w1774) -> ()  [unwired: 1 in, 2 out]
            }
          }
          n413 = Boolean To (0,1)(Boolean=w1455) -> (0, 1=w1581:i16[])
          n414 = Boolean Array To Number(Boolean array=w1455) -> (number=w1578:u32)
          n415 = Multiply(x=2.0, y=w1511) -> (x*y=w1519:dbl)
          n416 = Multiply(x=153.1621 ("y"), y=-1.0) -> (x*y=w1520:dbl)
          n417 = call "Warten13"("Count(mSec)"=u32 100) -> ()  [unwired: 1 out]
          n418 = Multiply(x=2.0 ("y"), y=w1478) -> (x*y=w1486:dbl)
          n419 = Multiply(x=153.1621 ("y"), y=-1.0) -> (x*y=w1488:dbl)
          n420 = To Long Integer(number=w1581) -> (32bit integer=w1580:i32[])
          n421 = Subtract(x=-237.2852 ("y"), y=w1508) -> (x-y=w1516:dbl)
          n422 = Greater?(x=w1578, y=u32 0) -> (0:w1576:bool)
          n423 = Or(x=w1576, y=w1451) -> (x .or. y?=w1457:bool)
          n424 = Divide(x=w1520, y=w1519) -> (x/y=w1513:dbl)
          n425 = Boolean To (0,1)(Boolean=w1446) -> (0, 1=w1593:i16[])
          n426 = Boolean Array To Number(Boolean array=w1446) -> (number=w1590:u32)
          n427 = Greater?(x=w1590, y=u32 0) -> (0:w1587:bool)
          n428 = Or(x=w1587, y=w1448) -> (x .or. y?=w1588:bool)
          n429 = case shown="True" w1588 {
            tunnel: w1458 -> [_ w1847]
            tunnel: w1449 -> [_ w1844]
            tunnel: w1585 -> [_ w1854]
            tunnel: w1584 -> [_ w1853]
            tunnel: w1506 -> [_ w1852]
            tunnel: w1447 -> [_ w1845]
            tunnel: w1446 -> [_ w1846]
            frame False {
            }
            frame True {
              n430 = local read "ZwangsDIO!"() -> (w1843:cluster{bool[]}[])
              n431 = for {
                tunnel: w1847 -> [w1869] mode=indexing
                tunnel: w1846 -> [w1868] mode=indexing
                tunnel: w1845 -> [w1867] mode=indexing
                tunnel: w1844 -> [w1866] mode=indexing
                tunnel: w1843 -> [w1865] mode=indexing
                tunnel: [w1855] -> w1842 mode=indexing
                n432 = Not(x=w1868) -> (.not. x?=w1871:bool)
                n433 = Unbundle(w1867) -> ("DIOsSPMod2B"=w1864:bool[][])
                n434 = Unbundle(w1866) -> (w1860:bool[])
                n435 = Unbundle(w1865) -> (w1859:bool[])
                n436 = Boolean To (0,1)(Boolean=w1871) -> (0, 1=w1870:i16)
                n437 = Not(x=w1860) -> (.not. x?=w1861:bool[])
                n438 = To Long Integer(number=w1870) -> (32bit integer=w1872:i32)
                n439 = Subtract(x=w1869, y=w1872) -> (x-y=w1863:i32)
                n440 = And(x=w1860, y=w1859) -> (x .and. y?=w1857:bool[])
                n441 = Index Array(array=w1864, index (row)=w1863) -> (element=w1862:bool[])  [unwired: 1 in]
                n442 = And(x=w1862, y=w1861) -> (x .and. y?=w1858:bool[])
                n443 = Or(x=w1858, y=w1857) -> (x .or. y?=w1856:bool[])
                n444 = Bundle(w1856) -> (w1855:cluster{bool[]})  [unwired: 1 in]
              }
              n445 = for {
                tunnel: w1842 -> [w1900] mode=indexing
                tunnel: w1854 -> [w1902] mode=indexing
                shift-right: [w1903] -> w1850
                shift-left: w1853 -> [w1904]
                n446 = Unbundle(w1900) -> (w1899:bool[])
                n447 = Unbundle(w1902) -> ("DIOsMod2BNr"=w1901:i32[])
                n448 = for {
                  tunnel: w1899 -> [w1906] mode=indexing
                  tunnel: w1901 -> [w1907] mode=indexing
                  shift-right: [w1905] -> w1903
                  shift-left: w1904 -> [w1908]
                  n449 = Replace Array Subset(array=w1908, new element=w1906, index=w1907) -> (w1905:bool[])
                }
              }
              n450 = Split 1D Array(array=w1850, index=32 ("Länge")) -> (first subarray=w1849:bool[], second subarray=w1848:bool[])
              n451 = xnode "Read/Write Control"("FPGA VI Reference In"=w1852, "Mod5/DIO"=w1849, "Mod6/DIO"=w1848) -> ()  [unwired: 1 in, 2 out]
            }
          }
          n452 = Subtract(x=-237.2852 ("y"), y=w1475) -> (x-y=w1483:dbl)
          n453 = Divide(x=w1488, y=w1486) -> (x/y=w1480:dbl)
          n454 = case shown="True" w1457 {
            tunnel: w1456 -> [_ w1606]
            tunnel: w1452 -> [_ w1607]
            tunnel: w1455 -> [_ w1609]
            tunnel: w1454 -> [_ w1608]
            frame False {
            }
            frame True {
              n455 = local read "ZwangsHorst!"() -> (w1605:cluster{dbl[]}[])
              n456 = for {
                tunnel: w1609 -> [w1629] mode=indexing
                tunnel: w1608 -> [w1626] mode=indexing
                tunnel: w1607 -> [w1632] mode=indexing
                tunnel: w1606 -> [w1630] mode=indexing
                tunnel: w1605 -> [w1631] mode=indexing
                shift-right: [w1610] -> w1603
                shift-left: dbl[] [] -> [w1612]
                n457 = Unbundle(w1630) -> ("HorstSPMod2B"=w1624:dbl[][])
                n458 = Unbundle(w1631) -> (w1615:dbl[])
                n459 = Unbundle(w1632) -> (w1619:bool[])
                n460 = Not(x=w1629) -> (.not. x?=w1628:bool)
                n461 = Not(x=w1619) -> (.not. x?=w1622:bool[])
                n462 = Boolean To (0,1)(Boolean=w1628) -> (0, 1=w1627:i16)
                n463 = To Long Integer(number=w1627) -> (32bit integer=w1625:i32)
                n464 = Boolean To (0,1)(Boolean=w1622) -> (0, 1=w1621:i16[])
                n465 = Boolean To (0,1)(Boolean=w1619) -> (0, 1=w1620:i16[])
                n466 = To Double Precision Float(number=w1621) -> (double precision float=w1617:dbl[])
                n467 = To Double Precision Float(number=w1620) -> (double precision float=w1616:dbl[])
                n468 = Subtract(x=w1626, y=w1625) -> (x-y=w1623:i32)
                n469 = Multiply(x=w1616, y=w1615) -> (x*y=w1613:dbl[])
                n470 = Index Array(array=w1624, index (row)=w1623) -> (element=w1618:dbl[])  [unwired: 1 in]
                n471 = Multiply(x=w1618, y=w1617) -> (x*y=w1614:dbl[])
                n472 = Add(x=w1614, y=w1613) -> (x+y=w1611:dbl[])
                n473 = Build Array (concatenate)(w1612, w1611) -> (w1610:dbl[])
              }
              "HorstSP" <- w1603
            }
          }
          n474 = Add(x=w1454, y=w1580) -> (x+y=w1579:i32[])
          n475 = Square(x=w1513) -> (x^2=w1518:dbl)
          n476 = Divide(x=w1516, y=w1511) -> (x/y=w1515:dbl)
          n477 = To Long Integer(number=w1593) -> (32bit integer=w1592:i32[])
          n478 = Square(x=w1480) -> (x^2=w1485:dbl)
          n479 = Divide(x=w1483, y=w1478) -> (x/y=w1482:dbl)
          n480 = Subtract(x=w1518, y=w1515) -> (x-y=w1514:dbl)
          n481 = Subtract(x=w1485, y=w1482) -> (x-y=w1481:dbl)
          n482 = Add(x=w1458, y=w1592) -> (x+y=w1591:i32[])
          n483 = Square Root(x=w1514) -> (sqrt(x)=w1512:dbl)
          n484 = Square Root(x=w1481) -> (sqrt(x)=w1479:dbl)
          n485 = Add(x=w1513, y=w1512) -> (x+y=w1510:dbl)
          n486 = local read "Methodenwechsel?"() -> (w1600:bool)
          n487 = Add(x=w1480, y=w1479) -> (x+y=w1477:dbl)
          n488 = To Fixed-Point(fixed-point type=fxp<+/-,16,4> 0.0 ("USetp [V]Mach1"), number=w1510) -> (fixed-point=w1507:fxp<+/-,16,4>)
          n489 = global read "gvbooleschRT.vi" "global stop RT"() -> (w1601:bool)
          n490 = To Fixed-Point(fixed-point type=fxp<+/-,16,4> 0.0 ("USetp [V]Mach1"), number=w1477) -> (fixed-point=w1468:fxp<+/-,16,4>)
          n491 = Or(x=w1600, y=w1601) -> (x .or. y?=w1602:bool)
          n492 = xnode "Read/Write Control"("FPGA VI Reference In"=w1506, "USetp[V]Mach1"=w1507, "USetp[V]Mach2"=w1468) -> ()  [unwired: 1 in, 2 out]
        }
        n493 = Equal?(x=w1444, y=0) -> (x = y?=w1442:bool)
        n494 = while "Zeit" {
          tunnel: w1442 -> [w1930]
          tunnel: [w1923] -> w1441
          tunnel: w1440 -> [w1929]
          tunnel: [w1916] -> w1439
          tunnel: w1436 -> [w1917]
          tunnel: w1417 -> [w1925]
          i -> [w1933]
          stop <- w1926 stop-if-true
          n495 = Equal?(x=w1933, y=0) -> (x = y?=w1931:bool)
          n496 = call "Warten3"("Count(mSec)"=u32 50) -> ()  [unwired: 1 out]
          n497 = And(x=w1930, y=w1931) -> (x .and. y?=w1935:bool)
          n498 = xnode "Elapsed Timer"("reset"=w1935) -> ("elapsed time (ms)"=w1938:i32)  [unwired: 2 in, 1 out]
          n499 = local read "Methodenwechsel?"() -> (w1928:bool)
          n500 = global read "gvbooleschRT.vi" "global stop RT"() -> (w1927:bool)
          n501 = Or(x=w1928, y=w1927) -> (x .or. y?=w1926:bool)
          n502 = To Double Precision Float(number=w1938) -> (double precision float=w1937:dbl)
          n503 = Divide(x=w1937, y=1000.0) -> (x/y=w1923:dbl)
          "Big Ben" <- w1923
          n504 = Subtract(x=w1923, y=w1929) -> (x-y=w1922:dbl)
          "Methodenzeit" <- w1922
          n505 = for {
            tunnel: w1925 -> [w1941] mode=indexing
            tunnel: w1922 -> [w1942]
            tunnel: [w1940] -> w1924 mode=indexing
            tunnel: [w1939] -> w1921 mode=indexing
            n506 = Quotient & Remainder(x=w1942, y=w1941) -> (x-y*floor(x/y)=w1940:dbl, floor(x/y)=w1939:dbl)
          }
          "Zykluszeiten 0, 1, 2A, 2B" <- w1924
          n507 = Build Array (concatenate)(w1923, w1922, w1924) -> (w1915:dbl[])
          n508 = To Long Integer(number=w1921) -> (32bit integer=w1920:i32[])
          "Zyklusnummern 0, 1, 2A, 2B" <- w1920
          n509 = local write "Big Ben, Methodenzeit, Zykluszeit0, Zykluszeit1, Zykluszeit2A, Zykluszeit2B"(w1915) -> ()
          n510 = Index Array(array=w1920, index=1 ("Index")) -> (element=w1918:i32)
          n511 = Add(x=w1918, y=w1917) -> (x+y=w1916:i32)
          "Zyklnum1ges" <- w1916
        }
        n512 = global read "gvbooleschRT.vi" "global stop RT"() -> (w1445:bool)
      }
      n513 = while {
        tunnel: w367 -> [w568]
        shift-right: [w566] -> _
        shift-left: _ -> [w569]
        tunnel: w375 -> [w573]
        shift-right: [w560] -> _
        shift-left: w341 -> [w572]
        tunnel: w373 -> [w571]
        tunnel: w372 -> [w570]
        tunnel: w374 -> [w567]
        tunnel: [w546] -> _
        i -> [w551]
        stop <- w574 stop-if-true
        n514 = for {
          tunnel: w573 -> [w592] mode=indexing
          tunnel: w572 -> [w603]
          tunnel: w571 -> [w602]
          tunnel: w570 -> [w601]
          tunnel: w569 -> [w600]
          tunnel: w568 -> [w593]
          tunnel: w567 -> [w599]
          tunnel: w567 -> [w580] mode=indexing
          tunnel: [w590] -> w566
          tunnel: [w579] -> w560
          tunnel: [w589] -> w559 mode=indexing
          tunnel: [w588] -> w558 mode=indexing
          tunnel: [w587] -> w557 mode=indexing
          tunnel: [w586] -> w556 mode=indexing
          tunnel: [w585] -> w555 mode=indexing
          tunnel: [w584] -> w554 mode=indexing
          tunnel: [w583] -> w553 mode=indexing
          tunnel: [w582] -> w552 mode=indexing
          n515 = local read "HorstSP"() -> (w579:dbl[])
          n516 = call "Warten7"("Count(mSec)"=u32 50) -> ()  [unwired: 1 out]
          n517 = for {
            tunnel: w579 -> [w615] mode=indexing
            tunnel: w603 -> [w618] mode=indexing
            tunnel: w602 -> [w617] mode=indexing
            tunnel: w601 -> [w616] mode=indexing
            tunnel: w600 -> [w614]
            tunnel: w593 -> [w613]
            tunnel: w599 -> [w612] mode=indexing
            tunnel: [w611] -> w594
            n518 = Not Equal?(x=w615, y=w618) -> (x != y?=w605:bool)
            n519 = local read "Zähler serielle Kommunikation"() -> (w609:i32)
            n520 = Quotient & Remainder(x=w609, y=10 ("Alle x Durchläufe Setpoints senden")) -> (x-y*floor(x/y)=w607:i32)  [unwired: 1 out]
            n521 = Equal?(x=w607, y=0) -> (x = y?=w610:bool)
            n522 = Or(x=w605, y=w610) -> (x .or. y?=w604:bool)
            n523 = case shown="True" w604 {
              tunnel: w617 -> [_ w625]
              tunnel: w616 -> [_ w633]
              tunnel: w615 -> [_ w634]
              tunnel: w614 -> [w619 w624]
              tunnel: w613 -> [_ w623]
              tunnel: w612 -> [_ w622]
              tunnel: [w619 w621] -> w611
              frame False {
              }
              frame True {
                n524 = Divide(x=w634, y=w633) -> (x/y=w627:dbl)
                n525 = call "Warten8"("Count(mSec)"=u32 50) -> ()  [unwired: 1 out]
                n526 = To Long Integer(number=w627) -> (32bit integer=w626:i32)
                n527 = Number To Hexadecimal String(1:i16 4 ("Breite (-)"), 2:w626) -> (0:w631:string)
                n528 = Concatenate Strings(w625, w631, "\r\n") -> (w629:string)
                n529 = call "serialwritefpga.vi"("FPGA VI Reference In"=w623, "Port"=w622, "String"=w629, "error in"=w624, "write"=TRUE) -> ("error out"=w621:errorcluster)  [unwired: 1 out]
              }
            }
          }
          n530 = Concatenate Strings(w592, "\r\n") -> (w596:string)
          n531 = call "serialwritefpga.vi"("FPGA VI Reference In"=w593, "Port"=w580, "String"=w596, "error in"=w594, "write"=TRUE) -> ("FPGA VI Reference Out"=w591:refnum<k20>, "error out"=w595:errorcluster)
          n532 = call "serialreadfpga2.vi"("error in"=w595, "FPGA VI Reference In"=w591) -> ("error out"=w590:errorcluster, "Port2"=w588:string, "Port1"=w589:string, "Port3"=w587:string, "Port7"=w583:string, "Port8"=w582:string, "Port4"=w586:string, "Port6"=w584:string, "Port5"=w585:string)  [unwired: 1 out]
        }
        n533 = xnode "Read/Write Control"("FPGA VI Reference In"=w568, "error in"=w566) -> ("FPGA VI Reference Out"=w546:refnum<k20>, "error out"=w578:errorcluster, "Error Out"=w577)
        n534 = Concatenate Strings(w552) -> (→"Port8":string)
        n535 = Concatenate Strings(w554) -> (→"Port6":string)
        n536 = Concatenate Strings(w555) -> (→"Port5":string)
        n537 = Concatenate Strings(w559) -> (w561:string)
        n538 = Concatenate Strings(w558) -> (w562:string)
        n539 = Concatenate Strings(w557) -> (w563:string)
        n540 = Concatenate Strings(w556) -> (w564:string)
        n541 = Concatenate Strings(w553) -> (→"Port7":string)
        n542 = Concatenate Strings(w561, w562, w563, w564) -> (→"RS-232":string)
        n543 = Merge Errors(w578, w577) -> (w575:errorcluster)
        n544 = global read "gvbooleschRT.vi" "global stop RT"() -> (w545:bool)
        n545 = Unbundle By Name(w575) -> ("status"=w576:bool)
        n546 = Or(x=w576, y=w545) -> (x .or. y?=w574:bool)
        "Zähler serielle Kommunikation" <- w551
      }
      n547 = while {
        tunnel: w371 -> [w499]
        tunnel: w372 -> [w500]
        shift-right: [w498] -> _
        shift-left: w341 -> [w501]
        shift-right: [w497] -> _
        shift-left: 0 ("Zähler serielle Kommunikation") -> [w496]
        stop <- w494 stop-if-true
        n548 = call "Warten10"("Count(mSec)"=u32 250) -> ()  [unwired: 1 out]
        n549 = local read "Zähler serielle Kommunikation"() -> (w497:i32)
        n550 = Not Equal?(x=w497, y=w496) -> (x != y?=w495:bool)
        n551 = case shown="True" w495 {
          tunnel: w501 -> [w502 w507]
          tunnel: w500 -> [_ w506]
          tunnel: w499 -> [_ w505]
          tunnel: [w502 w503] -> w498
          frame False {
          }
          frame True {
            n552 = local read "RS-232"() -> (w504:string)
            n553 = for {
              tunnel: w504 -> [w522]
              tunnel: w505 -> [w520] mode=indexing
              tunnel: w506 -> [w519] mode=indexing
              shift-right: [w517] -> w503
              shift-left: w507 -> [w516]
              i -> [w518]
              n554 = Match Pattern(string=w522, regular expression=w520) -> (match substring=w521:string, after substring=w512:string)  [unwired: 1 in, 2 out]
              n555 = Equal?(x=w521, y=w520) -> (x = y?=w510:bool)
              n556 = String Subset(string=w512, length (rest)=4 ("Länge (Rest)")) -> (substring=w511:string)  [unwired: 1 in]
              n557 = for {
                N: 4 -> [_]
                tunnel: w511 -> [w535]
                shift-right: [w523] -> w509
                shift-left: TRUE -> [w524]
                i -> [w534]
                n558 = String Subset(string=w535, offset (0)=w534, length (rest)=1 ("Länge (Rest)")) -> (substring=w530:string)
                n559 = Equal?(x=w530, y="0") -> (x = y?=w531:bool)
                n560 = Hexadecimal String To Number(string=w530, default (0uL)=0.0) -> (number=w528:dbl)  [unwired: 1 in, 1 out]
                n561 = Greater?(x=w528, y=0.0) -> (0:w526:bool)
                n562 = Or(x=w531, y=w526) -> (x .or. y?=w525:bool)
                n563 = And(x=w524, y=w525) -> (x .and. y?=w523:bool)
              }
              n564 = And(x=w510, y=w509) -> (x .and. y?=w508:bool)
              n565 = case shown="True" w508 {
                tunnel: w511 -> [_ w537]
                tunnel: w519 -> [_ w543]
                tunnel: w518 -> [_ w540]
                tunnel: [w536 w539] -> w517
                tunnel: w516 -> [w536 w538]
                frame False {
                }
                frame True {
                  n566 = Hexadecimal String To Number(string=w537, default (0uL)=0.0) -> (number=w542:dbl)  [unwired: 1 in, 1 out]
                  n567 = Multiply(x=w543, y=w542) -> (x*y=w541:dbl)
                  n568 = Replace Array Subset(array=w538, new element=w541, index=w540) -> (w539:dbl[])
                }
              }
            }
            "MWHorst" <- w503
          }
        }
        n569 = global read "gvbooleschRT.vi" "global stop RT"() -> (w494:bool)
      }
      n570 = while {
        stop <- w403 stop-if-true
        n571 = call "Warten17"("Count(mSec)"=u32 1000 ("Zu wartende ms")) -> ()  [unwired: 1 out]
        n572 = Get Date/Time In Seconds() -> (seconds since 1Jan1904=w405:timestamp)
        n573 = Format Date/Time String(time format string (%c)="%Y%m%d%H%M%S" ("Zeitformatierungs-String (%c)"), seconds (now)=w405) -> (date/time string=→"Datum/Zeit":string)  [unwired: 1 in]
        n574 = global read "gvbooleschRT.vi" "global stop RT"() -> (w403:bool)
      }
      n575 = while {
        tunnel: path "c:/fromcriocmd.txt" ("Dateipfad (Dialog verwenden)") -> [w414]
        tunnel: w338 -> [w415]
        stop <- w416 stop-if-true
        n576 = local read "Dateien fürs MS schicken?"() -> (w413:bool)
        n577 = global read "gvbooleschRT.vi" "global stop RT"() -> (w412:bool)
        n578 = Not(x=w412) -> (.not. x?=w411:bool)
        n579 = Boolean To (0,1)(Boolean=w411) -> (0, 1=w409:i16)
        n580 = case shown="True" w413 {
          tunnel: w414 -> [_ w423]
          tunnel: w415 -> [_ w422]
          tunnel: w414 -> [_ w419]
          frame False {
          }
          frame True {
            n581 = flat-sequence {
              tunnel: w419 -> [w425]
              tunnel: w423 -> [w426]
              tunnel: [w426] -> w418
              tunnel: [w425] -> w417
              tunnel: [w466] -> w420
              tunnel: w418 -> [w466]
              tunnel: w417 -> [w427]
              tunnel: [w473] -> w421
              tunnel: w420 -> [w478]
              tunnel: w422 -> [w486]
              tunnel: w421 -> [w482]
              frame #0 {
                n582 = call "Warten14"("Count(mSec)"=u32 1000 ("Zu wartende ms")) -> ()  [unwired: 1 out]
              }
              frame #1 {
                n583 = Open/Create/Replace File(file path (use dialog)=w427, operation (0:open)=T5."open" ("Operation (0:Öffnen)")) -> (refnum out=w431:refnum<file>)  [unwired: 4 in, 2 out]
                n584 = Read from Text File(file (use dialog)=w431) -> (refnum out=w432:refnum<file>)  [unwired: 3 in, 3 out]
                n585 = local read "Datum/Zeit"() -> (w454:string)
                n586 = Set File Position(offset (in bytes) (0)=i64 5 ("Offset (in Byte) (0)"), refnum=w432) -> (refnum out=w439:refnum<file>)  [unwired: 2 in, 1 out]
                n587 = local read "Zyklnum1ges"() -> (w456:i32)
                n588 = Write to Text File(file (use dialog)=w439, text=w454) -> (refnum out=w441:refnum<file>)  [unwired: 2 in, 2 out]
                n589 = Set File Position(offset (in bytes) (0)=i64 27 ("Offset (in Byte) (0)"), refnum=w441) -> (refnum out=w440:refnum<file>)  [unwired: 2 in, 1 out]
                n590 = Format Value(format string="%03d" ("Format-String"), value (0)=w456) -> (output string=w458:string)  [unwired: 1 in]
                n591 = String Length(string="Info") -> (length=w459:i32)
                n592 = Write to Text File(file (use dialog)=w440, text=w458) -> (refnum out=w442:refnum<file>)  [unwired: 2 in, 2 out]
                n593 = Subtract(x=100, y=w459) -> (x-y=w461:i32)
                n594 = Initialize Array(" ", w461) -> (w463:string[])
                n595 = Set File Position(offset (in bytes) (0)=i64 37 ("Offset (in Byte) (0)"), refnum=w442) -> (refnum out=w443:refnum<file>)  [unwired: 2 in, 1 out]
                n596 = Concatenate Strings("Info", w463) -> (w465:string)
                n597 = Write to Text File(file (use dialog)=w443, text=w465) -> (refnum out=w444:refnum<file>)  [unwired: 2 in, 2 out]
                n598 = Set File Position(offset (in bytes) (0)=i64 196 ("Offset (in Byte) (0)"), refnum=w444) -> (refnum out=w445:refnum<file>)  [unwired: 2 in, 1 out]
                n599 = case shown="0, Default" "wie wird gespeichert?" {
                  tunnel: ["Time" "Cycle" "all"] -> w453
                  tunnel: [i64 209 ("Größe (in Byte)") i64 210 ("Größe (in Byte)") i64 208 ("Größe (in Byte)")] -> w446
                  frame 0, Default {
                  }
                  frame 1 {
                  }
                  frame 2 {
                  }
                }
                n600 = Write to Text File(file (use dialog)=w445, text="Speicherlänge") -> (refnum out=w451:refnum<file>)  [unwired: 2 in, 2 out]
                n601 = Set File Position(offset (in bytes) (0)=i64 205 ("Offset (in Byte) (0)"), refnum=w451) -> (refnum out=w450:refnum<file>)  [unwired: 2 in, 1 out]
                n602 = Write to Text File(file (use dialog)=w450, text=w453) -> (refnum out=w452:refnum<file>)  [unwired: 2 in, 2 out]
                n603 = Set File Size(6:w446, 7:w452) -> (3:w447:refnum<file>)  [unwired: 1 in, 1 out]
                n604 = Set File Position(offset (in bytes) (0)=i64 0 ("Offset (in Byte) (0)"), refnum=w447) -> (refnum out=w437:refnum<file>)  [unwired: 2 in, 1 out]
                n605 = Read from Text File(file (use dialog)=w437) -> (refnum out=w448:refnum<file>, text=→"Text 6":string)  [unwired: 3 in, 2 out]
                n606 = Close File(refnum=w448) -> ()  [unwired: 1 in, 2 out]
              }
              frame #2 {
                n607 = call "Warten16"("Count(mSec)"=u32 500 ("Zu wartende ms")) -> ()  [unwired: 1 out]
                n608 = call <vilib>:"FTP Put File.vi"("remote port (21)"=u16 21, "password"="1" ("user"), "binary (F)"=TRUE, "user"="1", "local path"=w478, "remote path"="fromcriocmd.txt", "host"="10.1.1.101") -> ("error out"=w473:errorcluster)  [unwired: 3 in, 1 out]
              }
              frame #3 {
                n609 = call <vilib>:"FTP Put File.vi"("remote port (21)"=u16 21, "password"="1" ("user"), "binary (F)"=TRUE, "user"="1", "error in (no error)"=w482, "local path"=w486, "remote path"="fromcriordy.txt", "host"="10.1.1.101") -> ()  [unwired: 2 in, 2 out]
              }
            }
          }
        }
        n610 = To Unsigned Long Integer(number=w409) -> (unsigned 32bit integer=w408:u32)
        n611 = Multiply(x=u32 10000 ("Zu wartende ms"), y=w408) -> (x*y=w407:u32)
        n612 = call "Warten11"("Count(mSec)"=w407) -> ()  [unwired: 1 out]
        n613 = global read "gvbooleschRT.vi" "global stop RT"() -> (w416:bool)
      }
      n614 = while {
        shift-right: [w1984] -> w397
        shift-left: w400 -> [w1986]
        shift-right: [w1983] -> w396
        shift-left: w399 -> [w1985]
        shift-right: [w1987] -> _
        shift-left: 0 ("Zyklusnummer1") -> [w1989]
        tunnel: w337 -> [w1982]
        tunnel: w336 -> [w1981]
        stop <- w1991 stop-if-true
        n615 = call "Warten2"("Count(mSec)"=u32 500) -> ()  [unwired: 1 out]
        n616 = local read "Zyklnum1ges"() -> (w1987:i32)
        n617 = Greater?(x=w1987, y=w1989) -> (0:w1988:bool)
        n618 = case shown="True" w1988 {
          tunnel: w1987 -> [_ w1997]
          tunnel: w1986 -> [w1993 w2002]
          tunnel: w1985 -> [w1992 w2001]
          tunnel: [w1993 w1998] -> w1984
          tunnel: [w1992 w1996] -> w1983
          tunnel: w1982 -> [_ w1995]
          tunnel: w1981 -> [_ w1994]
          frame False {
          }
          frame True {
            n619 = flat-sequence {
              tunnel: w2002 -> [w2004]
              tunnel: w2001 -> [w2003]
              tunnel: [w2004] -> w2000
              tunnel: [w2003] -> w1999
              tunnel: w2000 -> [w2020]
              tunnel: w1999 -> [w2021]
              tunnel: [w2021] -> w1998
              tunnel: w1997 -> [w2015]
              tunnel: [w2013] -> w1996
              tunnel: w1995 -> [w2006]
              tunnel: w1994 -> [w2005]
              frame #0 {
                "aktuelle TDMS-Datei" <- w2003
              }
              frame #1 {
                n620 = TDMS Close(11:w2020) -> ()  [unwired: 1 in, 2 out]
                n621 = local read "Methodennummer"() -> (w2010:i32)
                n622 = Add(x=w2015, y=1) -> (x+y=w2017:i32)
                n623 = Number To Decimal String(number=w2010) -> (decimal integer string=w2009:string)  [unwired: 1 in]
                n624 = Number To Decimal String(number=w2017) -> (decimal integer string=w2007:string)  [unwired: 1 in]
                n625 = Concatenate Strings(w2006, "m", w2009, "z", w2007, ".tdms" ("String")) -> (w2016:string)
                n626 = Build Path(base path=w2005, name or relative path=w2016) -> (appended path=w2018:path)
                n627 = TDMS Open(10:T4."create" ("Operation (0:Öffnen)"), 11:w2018) -> (3:w2013:refnum<k34>)  [unwired: 4 in, 1 out]
              }
            }
          }
        }
        n628 = global read "gvbooleschRT.vi" "global stop RT"() -> (w1991:bool)
      }
    }
    frame #2 {
      n629 = TDMS Close(11:w2031) -> ()  [unwired: 1 in, 2 out]
      n630 = TDMS Close(11:w2030) -> ()  [unwired: 1 in, 2 out]
      n631 = xnode "Read/Write Control"("FPGA VI Reference In"=w2029, "global stop"=TRUE) -> ("FPGA VI Reference Out"=w2028:refnum<k20>)  [unwired: 1 in, 1 out]
      n632 = xnode "Close FPGA VI Reference"("FPGA VI Reference In"=w2028) -> ()  [unwired: 1 in, 1 out]
    }
  }
